vi "Least Pth Norm Complex Approximation-Compensate Channel Distortion.vi"() -> ()   [LabVIEW 2023]
doc: "Demonstrates a least pth norm complex approximation filter design. The designed filter compensates the channel distortion, both in the magnitude and phase, from some hardware devices. The goal of the compensation is to make the overall response have a flat passband magnitude response and an approximately linear phase.\n\nComplete the following steps to use this VI.\n1) Run the VI to design the bandpass finite impulse response (FIR) filter.\n2) View the graphs on the different tabs to observe the original measured channel response, designed filter magnitude, and phase response. The overall compensated channel response also is plotted.\n\n<B>Note:</B> The phase response is plotted in difference from linear phase, and the unit is in degree.\n\n3) Change the <B>Order</B>, <B>Group delay</B>, and <B>p</B>. Run the VI to redesign the filter and observe the design results."
uses:
  <vilib>/addons/Digital Filter Design/_LpNorm.llb/dfd_Lp Norm Filter Type.ctl
  <vilib>/addons/Digital Filter Design/_Objects.llb/DFD Phase Setting.ctl
  <vilib>/Utility/cursorutil.llb/Set Cursor (Icon Pict).vi
  <vilib>/addons/Digital Filter Design/Design.llb/DFD Least Pth Norm Design by IRLS.vi
  <vilib>/addons/Digital Filter Design/NI_DigFilterLicensed.lvlib
  <vilib>/Analysis/NI_AALPro.lvlib
panel:
  out "Status Str":string="Idle"
  out "Status LED":bool
  in  "?":T1(tab)
  out "Magnitude Response":cluster{dbl[], "magnitude":dbl[]}[](graph)
  out "Deviation From Linear Phase":cluster{dbl[], "magnitude":dbl[]}[](graph)
  out "Original Measured Channel Response":cluster{dbl[], dbl[]}[](graph)
  in  "p":i32=25
  in  "Order":cluster{"numerator":i32, "denominator":i32}={"numerator"=90, "denominator"=0}
  in  "Group Delay":dbl=15.0
  in  "Bandpass Specifications":T2(array[cluster])=[{"frequency point"=[{"frequency"=0.0, "magnitude"=0.0, "weight"=1.0, "phase"=0.0}]}, {"frequency point"=[{"frequency"=0.08333333333333334, "magnitude"=0.7291964977229365, "weight"=1.0, "phase"=-0.01642040201610384}, {"frequency"=0.08366700033366697, "magnitude"=0.7294776006658067, "weight"=1.0, "phase"=-0.015642400332134043}, {"frequency"=0.08400066733400066, "magnitude"=0.729821521109038, "weight"=1.0, "phase"=-0.014738419898844723}, {"frequency"=0.08433433433433435, "magnitude"=0.7302176778927697, "weight"=1.0, "phase"=-0.013743373051240626}, {"frequency"=0.08466800133466801, "magnitude"=0.7306554691620589, "weight"=1.0, "phase"=-0.01269217212432694}, {"frequency"=0.08500166833500167, "magnitude"=0.7311242586235973, "weight"=1.0, "phase"=-0.011619729453107519}, {"frequency"=0.08533533533533535, "magnitude"=0.7316133648627481, "weight"=1.0, "phase"=-0.010560957372586666}, {"frequency"=0.08566900233566904, "magnitude"=0.7321120537426865, "weight"=1.0, "phase"=-0.00955076821776979}, {"frequency"=0.0860026693360027, "magnitude"=0.7326095339186982, "weight"=1.0, "phase"=-0.00862407432366119}, {"frequency"=0.08633633633633633, "magnitude"=0.733094955508216, "weight"=1.0, "phase"=-0.007815788025265391}, {"frequency"=0.08667000333667002, "magnitude"=0.7335574119649325, "weight"=1.0, "phase"=-0.007160821643518167}, {"frequency"=0.08700367033700371, "magnitude"=0.733990132173198, "weight"=1.0, "phase"=-0.006679592999832229}, {"frequency"=0.08733733733733737, "magnitude"=0.7344025906833778, "weight"=1.0, "phase"=-0.006336255222158416}, {"frequency"=0.08767100433767103, "magnitude"=0.7348082615996662, "weight"=1.0, "phase"=-0.0060813110071700205}, {"frequency"=0.08800467133800471, "magnitude"=0.735220680155035, "weight"=1.0, "phase"=-0.005865263051539893}, {"frequency"=0.0883383383383384, "magnitude"=0.7356534427937741, "weight"=1.0, "phase"=-0.005638614051941548}, {"frequency"=0.08867200533867206, "magnitude"=0.7361202122718765, "weight"=1.0, "phase"=-0.0053518667050487245}, {"frequency"=0.08900567233900569, "magnitude"=0.7366347278394582, "weight"=1.0, "phase"=-0.004955523707534715}, {"frequency"=0.08933933933933938, "magnitude"=0.7372108205814925, "weight"=1.0, "phase"=-0.004400087756072146}, {"frequency"=0.08967300633967307, "magnitude"=0.7378624340133608, "weight"=1.0, "phase"=-0.003636061547334979}, {"frequency"=0.09000667334000673, "magnitude"=0.738603650013043, "weight"=1.0, "phase"=-0.0026139479515838726}, {"frequency"=0.09034034034034039, "magnitude"=0.7394429628053, "weight"=1.0, "phase"=-0.00130727564016353}, {"frequency"=0.09067400734067407, "magnitude"=0.7403672698363095, "weight"=1.0, "phase"=0.0002236847472032455}, {"frequency"=0.09100767434100776, "magnitude"=0.7413582649529322, "weight"=1.0, "phase"=0.0018982402282461397}, {"frequency"=0.09134134134134142, "magnitude"=0.7423974847865913, "weight"=1.0, "phase"=0.0036356978206948387}, {"frequency"=0.09167500834167505, "magnitude"=0.7434662792859068, "weight"=1.0, "phase"=0.005355364542279917}, {"frequency"=0.09200867534200874, "magnitude"=0.7445457913604945, "weight"=1.0, "phase"=0.006976547410731282}, {"frequency"=0.09234234234234243, "magnitude"=0.7456169458785842, "weight"=1.0, "phase"=0.008418553443778842}, {"frequency"=0.09267600934267609, "magnitude"=0.7466604482957828, "weight"=1.0, "phase"=0.009600689659152506}, {"frequency"=0.09300967634300975, "magnitude"=0.747656793207084, "weight"=1.0, "phase"=0.010442263074582181}, {"frequency"=0.09334334334334343, "magnitude"=0.7485862832307145, "weight"=1.0, "phase"=0.01086258136583651}, {"frequency"=0.09367701034367712, "magnitude"=0.7494340358118909, "weight"=1.0, "phase"=0.01080758126349246}, {"frequency"=0.09401067734401078, "magnitude"=0.7502033207758755, "weight"=1.0, "phase"=0.010320556929489966}, {"frequency"=0.09434434434434444, "magnitude"=0.7509016633673932, "weight"=1.0, "phase"=0.00946704597873893}, {"frequency"=0.0946780113446781, "magnitude"=0.751536690987375, "weight"=1.0, "phase"=0.008312586026149704}, {"frequency"=0.09501167834501179, "magnitude"=0.7521161195279792, "weight"=1.0, "phase"=0.006922714686632192}, {"frequency"=0.09534534534534544, "magnitude"=0.752647741160652, "weight"=1.0, "phase"=0.005362969575095633}, {"frequency"=0.0956790123456791, "magnitude"=0.7531394136376565, "weight"=1.0, "phase"=0.0036988883064501543}, {"frequency"=0.09601267934601279, "magnitude"=0.7535990511578299, "weight"=1.0, "phase"=0.0019960084956065494}, {"frequency"=0.09634634634634648, "magnitude"=0.7540346168388542, "weight"=1.0, "phase"=0.00031986775747405716}, {"frequency"=0.09668001334668014, "magnitude"=0.7544541166975602, "weight"=1.0, "phase"=-0.00126399716598935}, {"frequency"=0.0970136803470138, "magnitude"=0.7548632460642399, "weight"=1.0, "phase"=-0.0027053890336878883}, {"frequency"=0.09734734734734746, "magnitude"=0.7552593805388855, "weight"=1.0, "phase"=-0.004008541739136895}, {"frequency"=0.09768101434768114, "magnitude"=0.7556380338332156, "weight"=1.0, "phase"=-0.005189756855110916}, {"frequency"=0.0980146813480148, "magnitude"=0.7559947038644909, "weight"=1.0, "phase"=-0.006265335954384499}, {"frequency"=0.09834834834834846, "magnitude"=0.7563248750778283, "weight"=1.0, "phase"=-0.007251580609731301}, {"frequency"=0.09868201534868215, "magnitude"=0.7566240213122837, "weight"=1.0, "phase"=-0.008164792393925646}, {"frequency"=0.09901568234901584, "magnitude"=0.7568876092129782, "weight"=1.0, "phase"=-0.009021272879742526}, {"frequency"=0.0993493493493495, "magnitude"=0.7571111021899773, "weight"=1.0, "phase"=-0.009837323639955375}, {"frequency"=0.09968301634968316, "magnitude"=0.7572899649227769, "weight"=1.0, "phase"=-0.010629246247339186}, {"frequency"=0.10001668335001682, "magnitude"=0.7574196687623038, "weight"=1.0, "phase"=-0.011413341472922722}, {"frequency"=0.1003503503503505, "magnitude"=0.7574989854731671, "weight"=1.0, "phase"=-0.012198488335294577}, {"frequency"=0.10068401735068416, "magnitude"=0.7575380329833526, "weight"=1.0, "phase"=-0.012968003820737373}, {"frequency"=0.10101768435101782, "magnitude"=0.757549385635026, "weight"=1.0, "phase"=-0.013699705747336255}, {"frequency"=0.10135135135135151, "magnitude"=0.757545627611821, "weight"=1.0, "phase"=-0.014371411933176592}, {"frequency"=0.1016850183516852, "magnitude"=0.7575393458286972, "weight"=1.0, "phase"=-0.014960940196344419}, {"frequency"=0.10201868535201886, "magnitude"=0.7575431270020746, "weight"=1.0, "phase"=-0.015446108354925547}, {"frequency"=0.10235235235235252, "magnitude"=0.7575695589025218, "weight"=1.0, "phase"=-0.01580473422700579}, {"frequency"=0.10268601935268618, "magnitude"=0.7576312357911097, "weight"=1.0, "phase"=-0.01601463563067007}, {"frequency"=0.10301968635301986, "magnitude"=0.7577407680452105, "weight"=1.0, "phase"=-0.016053630384004647}, {"frequency"=0.10335335335335352, "magnitude"=0.7579107941667514, "weight"=1.0, "phase"=-0.015899538228420163}, {"frequency"=0.10368702035368718, "magnitude"=0.7581439480868885, "weight"=1.0, "phase"=-0.015540776351122831}, {"frequency"=0.10402068735402087, "magnitude"=0.7584092673045393, "weight"=1.0, "phase"=-0.015001192493993232}, {"frequency"=0.10435435435435456, "magnitude"=0.7586686932099818, "weight"=1.0, "phase"=-0.014312030150815502}, {"frequency"=0.10468802135468822, "magnitude"=0.7588840658506781, "weight"=1.0, "phase"=-0.013504532815374448}, {"frequency"=0.10502168835502187, "magnitude"=0.759017148989923, "weight"=1.0, "phase"=-0.012609943981453542}, {"frequency"=0.10535535535535553, "magnitude"=0.7590296936775417, "weight"=1.0, "phase"=-0.011659507142836922}, {"frequency"=0.10568902235568922, "magnitude"=0.7588835403489989, "weight"=1.0, "phase"=-0.010684465793309394}, {"frequency"=0.10602268935602288, "magnitude"=0.7585407591191804, "weight"=1.0, "phase"=-0.009716063426654653}, {"frequency"=0.10635635635635654, "magnitude"=0.7579638274268182, "weight"=1.0, "phase"=-0.008785543536657281}, {"frequency"=0.10669002335669023, "magnitude"=0.7571158500751093, "weight"=1.0, "phase"=-0.007924146927511755}, {"frequency"=0.10702369035702392, "magnitude"=0.7559841062871058, "weight"=1.0, "phase"=-0.007153519149495802}, {"frequency"=0.10735735735735757, "magnitude"=0.7546320301499954, "weight"=1.0, "phase"=-0.006464162750622782}, {"frequency"=0.10769102435769123, "magnitude"=0.7531378467913443, "weight"=1.0, "phase"=-0.005840273020128572}, {"frequency"=0.1080246913580249, "magnitude"=0.751578803079211, "weight"=1.0, "phase"=-0.005266045247247941}, {"frequency"=0.10835835835835858, "magnitude"=0.75003096166546, "weight"=1.0, "phase"=-0.004725674721217432}, {"frequency"=0.10869202535869224, "magnitude"=0.7485691524910209, "weight"=1.0, "phase"=-0.0042033567312727005}, {"frequency"=0.1090256923590259, "magnitude"=0.747267075522499, "weight"=1.0, "phase"=-0.003683286566649624}, {"frequency"=0.10935935935935959, "magnitude"=0.746197548757706, "weight"=1.0, "phase"=-0.003149659516583192}, {"frequency"=0.10969302635969327, "magnitude"=0.7454328970310171, "weight"=1.0, "phase"=-0.0025866708703092822}, {"frequency"=0.11002669336002693, "magnitude"=0.7450454672350842, "weight"=1.0, "phase"=-0.001978516626216953}, {"frequency"=0.1103603603603606, "magnitude"=0.7450774580732047, "weight"=1.0, "phase"=-0.0013111347269851858}, {"frequency"=0.11069402736069425, "magnitude"=0.7454750771451178, "weight"=1.0, "phase"=-0.0005759523096529051}, {"frequency"=0.11102769436102794, "magnitude"=0.7461663356684396, "weight"=1.0, "phase"=0.00023452495654474603}, {"frequency"=0.1113613613613616, "magnitude"=0.7470795280107462, "weight"=1.0, "phase"=0.0011277914023726243}, {"frequency"=0.11169502836169529, "magnitude"=0.7481427320752025, "weight"=1.0, "phase"=0.0021113413585955865}, {"frequency"=0.11202869536202895, "magnitude"=0.749283447281809, "weight"=1.0, "phase"=0.003192669155978489}, {"frequency"=0.1123623623623626, "magnitude"=0.7504283706287428, "weight"=1.0, "phase"=0.004379269125285967}, {"frequency"=0.11269602936269629, "magnitude"=0.7515033137097323, "weight"=1.0, "phase"=0.005678635597282655}, {"frequency"=0.11302969636302995, "magnitude"=0.7524332648354042, "weight"=1.0, "phase"=0.00709826290273341}, {"frequency"=0.11336336336336361, "magnitude"=0.7531426154406591, "weight"=1.0, "phase"=0.008645640535727361}, {"frequency"=0.1136970303636973, "magnitude"=0.7535820012382601, "weight"=1.0, "phase"=0.01031968524409188}, {"frequency"=0.11403069736403096, "magnitude"=0.7537834472908194, "weight"=1.0, "phase"=0.012093083021709417}, {"frequency"=0.11436436436436465, "magnitude"=0.7537950028511985, "weight"=1.0, "phase"=0.013933520165863245}, {"frequency"=0.1146980313646983, "magnitude"=0.7536650649271978, "weight"=1.0, "phase"=0.015808682973836197}, {"frequency"=0.11503169836503196, "magnitude"=0.7534421656477983, "weight"=1.0, "phase"=0.017686257742911327}, {"frequency"=0.11536536536536565, "magnitude"=0.75317482146964, "weight"=1.0, "phase"=0.019533930770371466}, {"frequency"=0.11569903236569931, "magnitude"=0.7529114448310957, "weight"=1.0, "phase"=0.021319388353499447}, {"frequency"=0.11603269936603297, "magnitude"=0.7527003182157362, "weight"=1.0, "phase"=0.023010316789578322}, {"frequency"=0.11636636636636666, "magnitude"=0.7525896302784149, "weight"=1.0, "phase"=0.024574402375890925}, {"frequency"=0.11670003336670032, "magnitude"=0.7526275620502375, "weight"=1.0, "phase"=0.025979336275783416}, {"frequency"=0.117033700367034, "magnitude"=0.7528469700766816, "weight"=1.0, "phase"=0.027199266918639387}, {"frequency"=0.11736736736736766, "magnitude"=0.7532349511268573, "weight"=1.0, "phase"=0.02822752962154551}, {"frequency"=0.11770103436770132, "magnitude"=0.7537702572793101, "weight"=1.0, "phase"=0.029061007061756072}, {"frequency"=0.11803470136803501, "magnitude"=0.7544317087878388, "weight"=1.0, "phase"=0.029696581916524467}, {"frequency"=0.11836836836836867, "magnitude"=0.7551981164450906, "weight"=1.0, "phase"=0.030131136863104535}, {"frequency"=0.11870203536870233, "magnitude"=0.7560482158426619, "weight"=1.0, "phase"=0.030361554578750116}, {"frequency"=0.11903570236903602, "magnitude"=0.7569606134289365, "weight"=1.0, "phase"=0.03038471774071483}, {"frequency"=0.11936936936936968, "magnitude"=0.75791374440808, "weight"=1.0, "phase"=0.03019750902625251}, {"frequency"=0.11970303636970336, "magnitude"=0.7588858426383042, "weight"=1.0, "phase"=0.02979681111261656}, {"frequency"=0.12003670337003702, "magnitude"=0.7598549237377591, "weight"=1.0, "phase"=0.029179516584385112}, {"frequency"=0.12037037037037068, "magnitude"=0.760799767015449, "weight"=1.0, "phase"=0.028352658384421803}, {"frequency"=0.12070403737070437, "magnitude"=0.761701802705473, "weight"=1.0, "phase"=0.027352532854794775}, {"frequency"=0.12103770437103803, "magnitude"=0.7625428113059467, "weight"=1.0, "phase"=0.02622068378784692}, {"frequency"=0.12137137137137169, "magnitude"=0.7633044390222347, "weight"=1.0, "phase"=0.02499865497592091}, {"frequency"=0.12170503837170538, "magnitude"=0.763968230946391, "weight"=1.0, "phase"=0.023727990211359407}, {"frequency"=0.12203870537203904, "magnitude"=0.7645156732675615, "weight"=1.0, "phase"=0.022450233286505084}, {"frequency"=0.12237237237237272, "magnitude"=0.7649282445346339, "weight"=1.0, "phase"=0.021206927993700386}, {"frequency"=0.12270603937270638, "magnitude"=0.7651874758978828, "weight"=1.0, "phase"=0.020039618125287983}, {"frequency"=0.12303970637304004, "magnitude"=0.7652750201436836, "weight"=1.0, "phase"=0.018989847473610544}, {"frequency"=0.12337337337337373, "magnitude"=0.7651727443448124, "weight"=1.0, "phase"=0.018099143076021118}, {"frequency"=0.12370704037370739, "magnitude"=0.7648750378917473, "weight"=1.0, "phase"=0.01739547656277618}, {"frequency"=0.12404070737404105, "magnitude"=0.7644108624232837, "weight"=1.0, "phase"=0.016868822350619705}, {"frequency"=0.12437437437437474, "magnitude"=0.7638152337984989, "weight"=1.0, "phase"=0.016502547184863436}, {"frequency"=0.1247080413747084, "magnitude"=0.7631231148491394, "weight"=1.0, "phase"=0.016280017810820002}, {"frequency"=0.12504170837504208, "magnitude"=0.7623693118813998, "weight"=1.0, "phase"=0.016184600973800922}, {"frequency"=0.12537537537537574, "magnitude"=0.7615884033021992, "weight"=1.0, "phase"=0.016199663419118826}, {"frequency"=0.1257090423757094, "magnitude"=0.7608147000421998, "weight"=1.0, "phase"=0.01630857189208479}, {"frequency"=0.12604270937604306, "magnitude"=0.7600822372374479, "weight"=1.0, "phase"=0.016494693138011662}, {"frequency"=0.12637637637637675, "magnitude"=0.7594247965425187, "weight"=1.0, "phase"=0.016741393902210966}, {"frequency"=0.12671004337671044, "magnitude"=0.7588759457608831, "weight"=1.0, "phase"=0.01703204768364519}, {"frequency"=0.1270437103770441, "magnitude"=0.7584608423530642, "weight"=1.0, "phase"=0.017354436479654956}, {"frequency"=0.12737737737737775, "magnitude"=0.7581820957925545, "weight"=1.0, "phase"=0.01770834697354684}, {"frequency"=0.1277110443777114, "magnitude"=0.758038649055317, "weight"=1.0, "phase"=0.018095590108574644}, {"frequency"=0.1280447113780451, "magnitude"=0.7580295918392452, "weight"=1.0, "phase"=0.018517976827991278}, {"frequency"=0.1283783783783788, "magnitude"=0.7581541574598288, "weight"=1.0, "phase"=0.018977318075050542}, {"frequency"=0.12871204537871245, "magnitude"=0.758411720146504, "weight"=1.0, "phase"=0.01947542479300579}, {"frequency"=0.1290457123790461, "magnitude"=0.7588017927246209, "weight"=1.0, "phase"=0.020014107925109936}, {"frequency"=0.12937937937937977, "magnitude"=0.7593240246700101, "weight"=1.0, "phase"=0.020595178414616777}, {"frequency"=0.12971304637971345, "magnitude"=0.7599782005250505, "weight"=1.0, "phase"=0.021220447204779225}, {"frequency"=0.13004671338004714, "magnitude"=0.7607642277028038, "weight"=1.0, "phase"=0.02189171669836809}, {"frequency"=0.1303803803803808, "magnitude"=0.7616762563851062, "weight"=1.0, "phase"=0.022606212271443882}, {"frequency"=0.13071404738071446, "magnitude"=0.7626928795648497, "weight"=1.0, "phase"=0.02334905001536902}, {"frequency"=0.13104771438104812, "magnitude"=0.7637899924581866, "weight"=1.0, "phase"=0.024103366347461908}, {"frequency"=0.1313813813813818, "magnitude"=0.7649432689104044, "weight"=1.0, "phase"=0.02485229768504027}, {"frequency"=0.13171504838171547, "magnitude"=0.7661281165964089, "weight"=1.0, "phase"=0.02557898044542206}, {"frequency"=0.13204871538204915, "magnitude"=0.7673196476006511, "weight"=1.0, "phase"=0.026266551045925457}, {"frequency"=0.1323823823823828, "magnitude"=0.768492664822771, "weight"=1.0, "phase"=0.026898145903868187}, {"frequency"=0.13271604938271647, "magnitude"=0.7696216647163575, "weight"=1.0, "phase"=0.027456901436568426}, {"frequency"=0.13304971638305013, "magnitude"=0.770680856886038, "weight"=1.0, "phase"=0.027925954061343905}, {"frequency"=0.13338338338338382, "magnitude"=0.7716442195449887, "weight"=1.0, "phase"=0.02828845657888923}, {"frequency"=0.1337170503837175, "magnitude"=0.7724938189234294, "weight"=1.0, "phase"=0.028534879091343557}, {"frequency"=0.13405071738405117, "magnitude"=0.7732329937236344, "weight"=1.0, "phase"=0.028674502851194772}, {"frequency"=0.13438438438438483, "magnitude"=0.773868596246044, "weight"=1.0, "phase"=0.028719590278690088}, {"frequency"=0.13471805138471848, "magnitude"=0.7744076143227507, "weight"=1.0, "phase"=0.028682403794075606}, {"frequency"=0.13505171838505217, "magnitude"=0.7748571530284708, "weight"=1.0, "phase"=0.028575205817598315}, {"frequency"=0.13538538538538586, "magnitude"=0.7752244174514789, "weight"=1.0, "phase"=0.02841025876950476}, {"frequency"=0.13571905238571952, "magnitude"=0.7755166966106241, "weight"=1.0, "phase"=0.028199825070041484}, {"frequency"=0.13605271938605318, "magnitude"=0.7757413485922225, "weight"=1.0, "phase"=0.027956167139454813}, {"frequency"=0.13638638638638684, "magnitude"=0.7759057869688721, "weight"=1.0, "phase"=0.027691547397991956}, {"frequency"=0.13672005338672052, "magnitude"=0.776017480607653, "weight"=1.0, "phase"=0.027418217720123206}, {"frequency"=0.13705372038705418, "magnitude"=0.7760884777587311, "weight"=1.0, "phase"=0.027144453398981527}, {"frequency"=0.13738738738738787, "magnitude"=0.7761422126005276, "weight"=1.0, "phase"=0.02686859494785021}, {"frequency"=0.13772105438772153, "magnitude"=0.7762038835409991, "weight"=1.0, "phase"=0.02658745687331021}, {"frequency"=0.1380547213880552, "magnitude"=0.7762987061026287, "weight"=1.0, "phase"=0.026297853681942263}, {"frequency"=0.13838838838838885, "magnitude"=0.7764519262776152, "weight"=1.0, "phase"=0.025996599880326876}, {"frequency"=0.13872205538872254, "magnitude"=0.7766888503112203, "weight"=1.0, "phase"=0.025680509975044785}, {"frequency"=0.13905572238905622, "magnitude"=0.7770348910233211, "weight"=1.0, "phase"=0.02534639847267628}, {"frequency"=0.13938938938938988, "magnitude"=0.7775156308826051, "weight"=1.0, "phase"=0.024991079879802314}, {"frequency"=0.13972305638972354, "magnitude"=0.7781569021987557, "weight"=1.0, "phase"=0.0246113687030034}, {"frequency"=0.1400567233900572, "magnitude"=0.7789848235248492, "weight"=1.0, "phase"=0.02420408589723766}, {"frequency"=0.14039039039039086, "magnitude"=0.7800061305427075, "weight"=1.0, "phase"=0.023768128762288843}, {"frequency"=0.14072405739072452, "magnitude"=0.7811795650745437, "weight"=1.0, "phase"=0.02330743640639965}, {"frequency"=0.14105772439105818, "magnitude"=0.7824563565035324, "weight"=1.0, "phase"=0.02282669841584628}, {"frequency"=0.14139139139139184, "magnitude"=0.783787198311825, "weight"=1.0, "phase"=0.02233060437690426}, {"frequency"=0.1417250583917255, "magnitude"=0.7851221459872021, "weight"=1.0, "phase"=0.02182384387584868}, {"frequency"=0.14205872539205916, "magnitude"=0.7864105772543553, "weight"=1.0, "phase"=0.021311106498955512}, {"frequency"=0.1423923923923928, "magnitude"=0.7876012167786005, "weight"=1.0, "phase"=0.020797081832500286}, {"frequency"=0.14272605939272645, "magnitude"=0.7886422275427034, "weight"=1.0, "phase"=0.020286459462758533}, {"frequency"=0.1430597263930601, "magnitude"=0.7894813707924199, "weight"=1.0, "phase"=0.019783928976005782}, {"frequency"=0.14339339339339374, "magnitude"=0.7900663336241841, "weight"=1.0, "phase"=0.019294162353024724}, {"frequency"=0.1437270603937274, "magnitude"=0.7903721297873525, "weight"=1.0, "phase"=0.01881694205332818}, {"frequency"=0.14406072739406106, "magnitude"=0.7904384644322694, "weight"=1.0, "phase"=0.018340509471393984}, {"frequency"=0.14439439439439472, "magnitude"=0.7903148153106312, "weight"=1.0, "phase"=0.01785144154599405}, {"frequency"=0.14472806139472838, "magnitude"=0.7900509258972148, "weight"=1.0, "phase"=0.017336315215900955}, {"frequency"=0.14506172839506204, "magnitude"=0.7896965978541807, "weight"=1.0, "phase"=0.016781707419886605}, {"frequency"=0.1453953953953957, "magnitude"=0.7893015459375388, "weight"=1.0, "phase"=0.01617419509672402}, {"frequency"=0.14572906239572936, "magnitude"=0.7889153156680115, "weight"=1.0, "phase"=0.01550035518518511}, {"frequency"=0.146062729396063, "magnitude"=0.7885872634877901, "weight"=1.0, "phase"=0.014746764624042452}, {"frequency"=0.14639639639639665, "magnitude"=0.7883665988554186, "weight"=1.0, "phase"=0.013900000352068176}, {"frequency"=0.1467300633967303, "magnitude"=0.7883023795503852, "weight"=1.0, "phase"=0.012946659083254985}, {"frequency"=0.14706373039706394, "magnitude"=0.7884176161425489, "weight"=1.0, "phase"=0.011878116921833382}, {"frequency"=0.1473973973973976, "magnitude"=0.7886754810078442, "weight"=1.0, "phase"=0.010696717238903197}, {"frequency"=0.14773106439773126, "magnitude"=0.7890308328248277, "weight"=1.0, "phase"=0.00940633560601567}, {"frequency"=0.14806473139806492, "magnitude"=0.789438466771787, "weight"=1.0, "phase"=0.008010847594721149}, {"frequency"=0.14839839839839858, "magnitude"=0.7898530284553761, "weight"=1.0, "phase"=0.006514128776570427}, {"frequency"=0.14873206539873224, "magnitude"=0.7902289796884825, "weight"=1.0, "phase"=0.004920054723113854}, {"frequency"=0.1490657323990659, "magnitude"=0.7905206165730275, "weight"=1.0, "phase"=0.003232501005902444}, {"frequency"=0.14939939939939956, "magnitude"=0.7906821403829216, "weight"=1.0, "phase"=0.001455343196486547}, {"frequency"=0.1497330663997332, "magnitude"=0.7906677815270303, "weight"=1.0, "phase"=-0.0004075431335828217}, {"frequency"=0.15006673340006685, "magnitude"=0.7904320804852738, "weight"=1.0, "phase"=-0.0023522401256306225}, {"frequency"=0.1504004004004005, "magnitude"=0.789952050916996, "weight"=1.0, "phase"=-0.004365865050543372}, {"frequency"=0.15073406740073414, "magnitude"=0.7892543280682364, "weight"=1.0, "phase"=-0.0064155333692217376}, {"frequency"=0.1510677344010678, "magnitude"=0.7883723804115088, "weight"=1.0, "phase"=-0.00846565416658529}, {"frequency"=0.15140140140140146, "magnitude"=0.7873396757681226, "weight"=1.0, "phase"=-0.010480636527553155}, {"frequency"=0.15173506840173512, "magnitude"=0.7861895411940636, "weight"=1.0, "phase"=-0.012424889537045125}, {"frequency"=0.15206873540206878, "magnitude"=0.7849550515057148, "weight"=1.0, "phase"=-0.014262822279980103}, {"frequency"=0.15240240240240244, "magnitude"=0.7836689463243245, "weight"=1.0, "phase"=-0.01595884384127766}, {"frequency"=0.1527360694027361, "magnitude"=0.7823635751765236, "weight"=1.0, "phase"=-0.01747736330585714}, {"frequency"=0.15306973640306976, "magnitude"=0.7810708699492893, "weight"=1.0, "phase"=-0.018782789758637897}, {"frequency"=0.1534034034034034, "magnitude"=0.7798223046093645, "weight"=1.0, "phase"=-0.01983959159961257}, {"frequency"=0.15373707040373705, "magnitude"=0.7786416306035427, "weight"=1.0, "phase"=-0.020623346504556217}, {"frequency"=0.1540707374040707, "magnitude"=0.777536480412578, "weight"=1.0, "phase"=-0.021133734673326687}, {"frequency"=0.15440440440440434, "magnitude"=0.7765123636812452, "weight"=1.0, "phase"=-0.021373594133709428}, {"frequency"=0.154738071404738, "magnitude"=0.775574775149403, "weight"=1.0, "phase"=-0.02134576291348922}, {"frequency"=0.15507173840507166, "magnitude"=0.7747292070728129, "weight"=1.0, "phase"=-0.021053079040451728}, {"frequency"=0.15540540540540532, "magnitude"=0.7739811624124456, "weight"=1.0, "phase"=-0.02049838054238151}, {"frequency"=0.15573907240573898, "magnitude"=0.7733361688179615, "weight"=1.0, "phase"=-0.019684505447064016}, {"frequency"=0.15607273940607264, "magnitude"=0.7727997934393749, "weight"=1.0, "phase"=-0.018614291782284464}, {"frequency"=0.1564064064064063, "magnitude"=0.7723776586098376, "weight"=1.0, "phase"=-0.017290577575827637}, {"frequency"=0.15674007340673995, "magnitude"=0.7720754381861281, "weight"=1.0, "phase"=-0.01571630295716475}, {"frequency"=0.1570737404070736, "magnitude"=0.7718955220278957, "weight"=1.0, "phase"=-0.013911411476722702}, {"frequency"=0.15740740740740725, "magnitude"=0.7718332930025463, "weight"=1.0, "phase"=-0.011931723652305548}, {"frequency"=0.1577410744077409, "magnitude"=0.771883344582029, "weight"=1.0, "phase"=-0.009837610392309903}, {"frequency"=0.15807474140807454, "magnitude"=0.7720403686742942, "weight"=1.0, "phase"=-0.0076894426051330456}, {"frequency"=0.1584084084084082, "magnitude"=0.7722991405081276, "weight"=1.0, "phase"=-0.0055475911991713645}, {"frequency"=0.15874207540874186, "magnitude"=0.7726545044106865, "weight"=1.0, "phase"=-0.0034724270828223602}, {"frequency"=0.15907574240907552, "magnitude"=0.773101360419999, "weight"=1.0, "phase"=-0.0015243211644822008}, {"frequency"=0.15940940940940918, "magnitude"=0.7736346516830314, "weight"=1.0, "phase"=0.0002363556474513917}, {"frequency"=0.15974307640974283, "magnitude"=0.7742493525975808, "weight"=1.0, "phase"=0.0017492324445820273}, {"frequency"=0.1600767434100765, "magnitude"=0.7749404253858766, "weight"=1.0, "phase"=0.0029541495560845288}, {"frequency"=0.16041041041041015, "magnitude"=0.7756980246918873, "weight"=1.0, "phase"=0.003822409834033591}, {"frequency"=0.16074407741074379, "magnitude"=0.7765023576223046, "weight"=1.0, "phase"=0.0043898853640069735}, {"frequency"=0.16107774441107744, "magnitude"=0.7773322689210734, "weight"=1.0, "phase"=0.004700374336808588}, {"frequency"=0.1614114114114111, "magnitude"=0.7781664297395946, "weight"=1.0, "phase"=0.004797674943243901}, {"frequency"=0.16174507841174474, "magnitude"=0.7789833289821583, "weight"=1.0, "phase"=0.004725585374116825}, {"frequency"=0.1620787454120784, "magnitude"=0.7797612764422021, "weight"=1.0, "phase"=0.004527903820232382}, {"frequency"=0.16241241241241205, "magnitude"=0.7804784179880816, "weight"=1.0, "phase"=0.004248428472394927}, {"frequency"=0.16274607941274571, "magnitude"=0.7811127630366153, "weight"=1.0, "phase"=0.003930957521409484}, {"frequency"=0.16307974641307937, "magnitude"=0.7816422245033707, "weight"=1.0, "phase"=0.0036192891580801856}, {"frequency"=0.16341341341341303, "magnitude"=0.7820447957730101, "weight"=1.0, "phase"=0.003357068641201222}, {"frequency"=0.1637470804137467, "magnitude"=0.7823151671612101, "weight"=1.0, "phase"=0.0031674603763960363}, {"frequency"=0.16408074741408035, "magnitude"=0.7824814491427057, "weight"=1.0, "phase"=0.0030327421129194843}, {"frequency"=0.16441441441441398, "magnitude"=0.7825758572218253, "weight"=1.0, "phase"=0.002930335300654674}, {"frequency"=0.16474808141474764, "magnitude"=0.782630692236983, "weight"=1.0, "phase"=0.0028376613894851577}, {"frequency"=0.1650817484150813, "magnitude"=0.7826782943728545, "weight"=1.0, "phase"=0.0027321418292947097}, {"frequency"=0.16541541541541493, "magnitude"=0.7827510238280951, "weight"=1.0, "phase"=0.0025911980699666604}, {"frequency"=0.1657490824157486, "magnitude"=0.782881268222221, "weight"=1.0, "phase"=0.002392251561384562}, {"frequency"=0.16608274941608225, "magnitude"=0.7831014768046424, "weight"=1.0, "phase"=0.0021127237534319665}, {"frequency"=0.1664164164164159, "magnitude"=0.7834442216012613, "weight"=1.0, "phase"=0.0017300360959928707}, {"frequency"=0.16675008341674957, "magnitude"=0.7839420974132115, "weight"=1.0, "phase"=0.0012217256976476687}, {"frequency"=0.16708375041708323, "magnitude"=0.7846051909938612, "weight"=1.0, "phase"=0.0005793243693956729}, {"frequency"=0.1674174174174169, "magnitude"=0.7853994173812051, "weight"=1.0, "phase"=-0.00017845628381407685}, {"frequency"=0.16775108441775055, "magnitude"=0.786285451511054, "weight"=1.0, "phase"=-0.0010297818721944907}, {"frequency"=0.16808475141808418, "magnitude"=0.7872236953163515, "weight"=1.0, "phase"=-0.001952818005959589}, {"frequency"=0.16841841841841784, "magnitude"=0.7881742040127784, "weight"=1.0, "phase"=-0.002925730295322504}, {"frequency"=0.16875208541875147, "magnitude"=0.7890966522953946, "weight"=1.0, "phase"=-0.00392668435049659}, {"frequency"=0.16908575241908513, "magnitude"=0.7899503413773119, "weight"=1.0, "phase"=-0.004933845781695201}, {"frequency"=0.1694194194194188, "magnitude"=0.7906942478624417, "weight"=1.0, "phase"=-0.005925380199132135}, {"frequency"=0.16975308641975245, "magnitude"=0.791287115327246, "weight"=1.0, "phase"=-0.0068794532130207475}, {"frequency"=0.1700867534200861, "magnitude"=0.7916877718956166, "weight"=1.0, "phase"=-0.0077743023941321265}, {"frequency"=0.17042042042041977, "magnitude"=0.791875199175099, "weight"=1.0, "phase"=-0.008596067512712136}, {"frequency"=0.17075408742075343, "magnitude"=0.7918665924579612, "weight"=1.0, "phase"=-0.009345820596954768}, {"frequency"=0.1710877544210871, "magnitude"=0.7916836670874443, "weight"=1.0, "phase"=-0.010026292763876565}, {"frequency"=0.17142142142142075, "magnitude"=0.7913483487483515, "weight"=1.0, "phase"=-0.010640215130492958}, {"frequency"=0.17175508842175438, "magnitude"=0.7908826833003659, "weight"=1.0, "phase"=-0.011190318813820044}, {"frequency"=0.17208875542208804, "magnitude"=0.7903087584550132, "weight"=1.0, "phase"=-0.011679334930873253}, {"frequency"=0.17242242242242167, "magnitude"=0.7896486376369792, "weight"=1.0, "phase"=-0.012109994598669349}, {"frequency"=0.17275608942275533, "magnitude"=0.7889243062026096, "weight"=1.0, "phase"=-0.012485028934223319}, {"frequency"=0.173089756423089, "magnitude"=0.7881576300484647, "weight"=1.0, "phase"=-0.012807169054551815}, {"frequency"=0.17342342342342265, "magnitude"=0.7873702882046637, "weight"=1.0, "phase"=-0.01307916245619778}, {"frequency"=0.1737570904237563, "magnitude"=0.7865799668699145, "weight"=1.0, "phase"=-0.013305395712733259}, {"frequency"=0.17409075742408997, "magnitude"=0.785797187968144, "weight"=1.0, "phase"=-0.013493269211688586}, {"frequency"=0.17442442442442363, "magnitude"=0.7850316370370765, "weight"=1.0, "phase"=-0.01365050706740134}, {"frequency"=0.1747580914247573, "magnitude"=0.7842929254919077, "weight"=1.0, "phase"=-0.013784833394208773}, {"frequency"=0.17509175842509092, "magnitude"=0.78359059621545, "weight"=1.0, "phase"=-0.013903972306448242}, {"frequency"=0.17542542542542458, "magnitude"=0.7829341314503409, "weight"=1.0, "phase"=-0.014015647918457108}, {"frequency"=0.17575909242575824, "magnitude"=0.7823329629570455, "weight"=1.0, "phase"=-0.014127584344572619}, {"frequency"=0.17609275942609187, "magnitude"=0.7817964844107049, "weight"=1.0, "phase"=-0.014247505699132135}, {"frequency"=0.17642642642642553, "magnitude"=0.7813340660214041, "weight"=1.0, "phase"=-0.014383136096472904}, {"frequency"=0.1767600934267592, "magnitude"=0.7809549212888665, "weight"=1.0, "phase"=-0.014542192217718353}, {"frequency"=0.17709376042709285, "magnitude"=0.7806545489148162, "weight"=1.0, "phase"=-0.014731710355687544}, {"frequency"=0.1774274274274265, "magnitude"=0.7804039618813459, "weight"=1.0, "phase"=-0.01495750933809159}, {"frequency"=0.17776109442776017, "magnitude"=0.780171729007459, "weight"=1.0, "phase"=-0.015225281606331409}, {"frequency"=0.17809476142809383, "magnitude"=0.7799265018414864, "weight"=1.0, "phase"=-0.015540719601807917}, {"frequency"=0.1784284284284275, "magnitude"=0.7796370124313223, "weight"=1.0, "phase"=-0.015909515765922144}, {"frequency"=0.17876209542876112, "magnitude"=0.7792720961989618, "weight"=1.0, "phase"=-0.01633736254007523}, {"frequency"=0.17909576242909478, "magnitude"=0.7788007397033747, "weight"=1.0, "phase"=-0.016829952365667866}, {"frequency"=0.17942942942942844, "magnitude"=0.7781921529576563, "weight"=1.0, "phase"=-0.017392977684101307}, {"frequency"=0.17976309642976207, "magnitude"=0.7774158657666472, "weight"=1.0, "phase"=-0.018032130936776358}, {"frequency"=0.18009676343009573, "magnitude"=0.7764421599476653, "weight"=1.0, "phase"=-0.018752879901885122}, {"frequency"=0.1804304304304294, "magnitude"=0.7752680846308073, "weight"=1.0, "phase"=-0.019541816438331083}, {"frequency"=0.18076409743076305, "magnitude"=0.7739364963197164, "weight"=1.0, "phase"=-0.020352659974254617}, {"frequency"=0.1810977644310967, "magnitude"=0.7724944530038845, "weight"=1.0, "phase"=-0.02113583298286492}, {"frequency"=0.18143143143143037, "magnitude"=0.7709884550783581, "weight"=1.0, "phase"=-0.02184175793737153}, {"frequency"=0.18176509843176403, "magnitude"=0.769464343942917, "weight"=1.0, "phase"=-0.022420857310983644}, {"frequency"=0.1820987654320977, "magnitude"=0.7679672565700568, "weight"=1.0, "phase"=-0.02282355357691057}, {"frequency"=0.18243243243243132, "magnitude"=0.7665416339934503, "weight"=1.0, "phase"=-0.023000269208361623}, {"frequency"=0.18276609943276498, "magnitude"=0.7652312815911121, "weight"=1.0, "phase"=-0.02290142667854622}, {"frequency"=0.18309976643309864, "magnitude"=0.7640794792196335, "weight"=1.0, "phase"=-0.022477448460673455}, {"frequency"=0.18343343343343227, "magnitude"=0.763128816455821, "weight"=1.0, "phase"=-0.021679256355123466}, {"frequency"=0.18376710043376593, "magnitude"=0.762396763376875, "weight"=1.0, "phase"=-0.02049640529040564}, {"frequency"=0.1841007674340996, "magnitude"=0.761858750809536, "weight"=1.0, "phase"=-0.018983936028781567}, {"frequency"=0.18443443443443325, "magnitude"=0.7614865763417724, "weight"=1.0, "phase"=-0.017203232636939902}, {"frequency"=0.1847681014347669, "magnitude"=0.7612523880355236, "weight"=1.0, "phase"=-0.01521567918156963}, {"frequency"=0.18510176843510057, "magnitude"=0.761128573548382, "weight"=1.0, "phase"=-0.013082659729359403}, {"frequency"=0.18543543543543423, "magnitude"=0.7610876701358569, "weight"=1.0, "phase"=-0.010865558346998205}, {"frequency"=0.18576910243576789, "magnitude"=0.7611022949262735, "weight"=1.0, "phase"=-0.008625759101174468}, {"frequency"=0.18610276943610152, "magnitude"=0.7611450951049089, "weight"=1.0, "phase"=-0.00642464605857751}, {"frequency"=0.18643643643643518, "magnitude"=0.7611887178255707, "weight"=1.0, "phase"=-0.004323603285895872}, {"frequency"=0.18677010343676884, "magnitude"=0.7612061098859204, "weight"=1.0, "phase"=-0.0023835745623049798}, {"frequency"=0.18710377043710247, "magnitude"=0.7611923755147278, "weight"=1.0, "phase"=-0.0006340398028947813}, {"frequency"=0.18743743743743613, "magnitude"=0.7611791869901544, "weight"=1.0, "phase"=0.0009474370951433331}, {"frequency"=0.1877711044377698, "magnitude"=0.7612016341731817, "weight"=1.0, "phase"=0.002388147338868829}, {"frequency"=0.18810477143810345, "magnitude"=0.7612948218792615, "weight"=1.0, "phase"=0.003715382135341061}, {"frequency"=0.1884384384384371, "magnitude"=0.7614939189492174, "weight"=1.0, "phase"=0.0049564326916193835}, {"frequency"=0.18877210543877077, "magnitude"=0.7618342398731551, "weight"=1.0, "phase"=0.00613859021476304}, {"frequency"=0.18910577243910442, "magnitude"=0.7623513593848505, "weight"=1.0, "phase"=0.007289145911831607}, {"frequency"=0.18943943943943806, "magnitude"=0.7630812608276689, "weight"=1.0, "phase"=0.008435390989884217}, {"frequency"=0.18977310643977172, "magnitude"=0.7640605196125, "weight"=1.0, "phase"=0.009604616655980336}, {"frequency"=0.19010677344010538, "magnitude"=0.7653260205824789, "weight"=1.0, "phase"=0.01082378521657823}, {"frequency"=0.19044044044043903, "magnitude"=0.7668822715457455, "weight"=1.0, "phase"=0.012098089227209119}, {"frequency"=0.19077410744077267, "magnitude"=0.7686805085527719, "weight"=1.0, "phase"=0.01339775242870167}, {"frequency"=0.19110777444110633, "magnitude"=0.7706666386269962, "weight"=1.0, "phase"=0.014689842529357566}, {"frequency"=0.19144144144143999, "magnitude"=0.7727857390054443, "weight"=1.0, "phase"=0.01594142723747838}, {"frequency"=0.19177510844177365, "magnitude"=0.7749818183568336, "weight"=1.0, "phase"=0.0171195742613659}, {"frequency"=0.1921087754421073, "magnitude"=0.7771976551248649, "weight"=1.0, "phase"=0.01819135130932159}, {"frequency"=0.19244244244244096, "magnitude"=0.7793747170298282, "weight"=1.0, "phase"=0.019123826089647245}, {"frequency"=0.19277610944277462, "magnitude"=0.7814531665522428, "weight"=1.0, "phase"=0.019884066310644544}, {"frequency"=0.19310977644310826, "magnitude"=0.7833719575077734, "weight"=1.0, "phase"=0.02043913968061506}, {"frequency"=0.19344344344344191, "magnitude"=0.7850695071072663, "weight"=1.0, "phase"=0.02075650639096871}, {"frequency"=0.19377711044377557, "magnitude"=0.7865130996553082, "weight"=1.0, "phase"=0.020827750839941817}, {"frequency"=0.19411077744410923, "magnitude"=0.7877164340277312, "weight"=1.0, "phase"=0.02068218450278858}, {"frequency"=0.19444444444444287, "magnitude"=0.7886979140195214, "weight"=1.0, "phase"=0.02035240361412316}, {"frequency"=0.19477811144477652, "magnitude"=0.7894765420990544, "weight"=1.0, "phase"=0.019871004408559934}, {"frequency"=0.19511177844511018, "magnitude"=0.790071815637584, "weight"=1.0, "phase"=0.01927058312071317}, {"frequency"=0.19544544544544384, "magnitude"=0.7905036305838448, "weight"=1.0, "phase"=0.018583735985196914}, {"frequency"=0.1957791124457775, "magnitude"=0.7907921935484516, "weight"=1.0, "phase"=0.017843059236625547}, {"frequency"=0.19611277944611116, "magnitude"=0.7909579430794995, "weight"=1.0, "phase"=0.017081149109613225}, {"frequency"=0.19644644644644482, "magnitude"=0.7910214807392825, "weight"=1.0, "phase"=0.016330601838774328}, {"frequency"=0.19678011344677845, "magnitude"=0.7910034321248022, "weight"=1.0, "phase"=0.015623727919529817}, {"frequency"=0.1971137804471121, "magnitude"=0.7909198848491026, "weight"=1.0, "phase"=0.014976488482277062}, {"frequency"=0.19744744744744577, "magnitude"=0.7907799583133622, "weight"=1.0, "phase"=0.014379949986428331}, {"frequency"=0.19778111444777943, "magnitude"=0.7905921991227813, "weight"=1.0, "phase"=0.013823088801961925}, {"frequency"=0.19811478144811306, "magnitude"=0.7903651573287301, "weight"=1.0, "phase"=0.01329488129885581}, {"frequency"=0.19844844844844672, "magnitude"=0.7901073770356786, "weight"=1.0, "phase"=0.012784303847088507}, {"frequency"=0.19878211544878038, "magnitude"=0.7898273888597787, "weight"=1.0, "phase"=0.012280332816637984}, {"frequency"=0.19911578244911404, "magnitude"=0.7895337042390476, "weight"=1.0, "phase"=0.01177194457748254}, {"frequency"=0.1994494494494477, "magnitude"=0.7892348115891015, "weight"=1.0, "phase"=0.011248115499600364}, {"frequency"=0.19978311644978136, "magnitude"=0.788939174294086, "weight"=1.0, "phase"=0.010697821952969755}, {"frequency"=0.20011678345011502, "magnitude"=0.788655244788933, "weight"=1.0, "phase"=0.010110321268279154}, {"frequency"=0.20045045045044865, "magnitude"=0.7883922131192629, "weight"=1.0, "phase"=0.009489869818689045}, {"frequency"=0.2007841174507823, "magnitude"=0.7881603753191809, "weight"=1.0, "phase"=0.00886296246810736}, {"frequency"=0.20111778445111597, "magnitude"=0.787970100399019, "weight"=1.0, "phase"=0.008257893703417785}, {"frequency"=0.20145145145144963, "magnitude"=0.7878317484848482, "weight"=1.0, "phase"=0.007702958011503891}, {"frequency"=0.20178511845178326, "magnitude"=0.7877556831411308, "weight"=1.0, "phase"=0.007226449879249475}, {"frequency"=0.20211878545211692, "magnitude"=0.7877522864234318, "weight"=1.0, "phase"=0.006856663793538442}, {"frequency"=0.20245245245245058, "magnitude"=0.7878319766862969, "weight"=1.0, "phase"=0.006621894241254145}, {"frequency"=0.20278611945278424, "magnitude"=0.7880052291896679, "weight"=1.0, "phase"=0.0065504357092806}, {"frequency"=0.2031197864531179, "magnitude"=0.7882825995686535, "weight"=1.0, "phase"=0.0066705826845014915}, {"frequency"=0.20345345345345156, "magnitude"=0.7886744834495161, "weight"=1.0, "phase"=0.007010054495130924}, {"frequency"=0.20378712045378522, "magnitude"=0.7891780764666628, "weight"=1.0, "phase"=0.007567861452006386}, {"frequency"=0.20412078745411885, "magnitude"=0.7897713733762997, "weight"=1.0, "phase"=0.008301563782258436}, {"frequency"=0.2044544544544525, "magnitude"=0.7904308015314588, "weight"=1.0, "phase"=0.009165490094484308}, {"frequency"=0.20478812145478617, "magnitude"=0.7911326715306077, "weight"=1.0, "phase"=0.010113968997281342}, {"frequency"=0.20512178845511983, "magnitude"=0.791853144261536, "weight"=1.0, "phase"=0.011101329099246882}, {"frequency"=0.20545545545545346, "magnitude"=0.7925682121202886, "weight"=1.0, "phase"=0.012081899008978159}, {"frequency"=0.20578912245578712, "magnitude"=0.7932536946422946, "weight"=1.0, "phase"=0.013010007335072737}, {"frequency"=0.20612278945612078, "magnitude"=0.7938852488130205, "weight"=1.0, "phase"=0.01383998268612785}, {"frequency"=0.20645645645645444, "magnitude"=0.7944383943186978, "weight"=1.0, "phase"=0.014526153670740838}, {"frequency"=0.2067901234567881, "magnitude"=0.794888872738692, "weight"=1.0, "phase"=0.015023255141737302}, {"frequency"=0.20712379045712176, "magnitude"=0.7952273056477532, "weight"=1.0, "phase"=0.01530501958997843}, {"frequency"=0.20745745745745542, "magnitude"=0.795465364283819, "weight"=1.0, "phase"=0.015371891060834808}, {"frequency"=0.20779112445778905, "magnitude"=0.7956164072774161, "weight"=1.0, "phase"=0.015226319012002665}, {"frequency"=0.2081247914581227, "magnitude"=0.7956938772257235, "weight"=1.0, "phase"=0.014870752901178341}, {"frequency"=0.20845845845845637, "magnitude"=0.7957112735314166, "weight"=1.0, "phase"=0.014307642186058178}, {"frequency"=0.20879212545879003, "magnitude"=0.7956821297208004, "weight"=1.0, "phase"=0.013539436324338405}, {"frequency"=0.20912579245912366, "magnitude"=0.7956199953124437, "weight"=1.0, "phase"=0.012568584773715474}, {"frequency"=0.20945945945945732, "magnitude"=0.7955384222785261, "weight"=1.0, "phase"=0.011397536991885504}, {"frequency"=0.20979312645979098, "magnitude"=0.7954509561185107, "weight"=1.0, "phase"=0.010028742436544835}, {"frequency"=0.21012679346012464, "magnitude"=0.7953710208410371, "weight"=1.0, "phase"=0.008465279155193572}, {"frequency"=0.2104604604604583, "magnitude"=0.7953071713201773, "weight"=1.0, "phase"=0.006737816887710801}, {"frequency"=0.21079412746079196, "magnitude"=0.7952613058024552, "weight"=1.0, "phase"=0.004914808304224638}, {"frequency"=0.21112779446112562, "magnitude"=0.795234843255541, "weight"=1.0, "phase"=0.00306743625693795}, {"frequency"=0.21146146146145925, "magnitude"=0.7952292049746124, "weight"=1.0, "phase"=0.00126688359805327}, {"frequency"=0.2117951284617929, "magnitude"=0.7952458153019017, "weight"=1.0, "phase"=-0.00041566682022653456}, {"frequency"=0.21212879546212657, "magnitude"=0.7952861023983617, "weight"=1.0, "phase"=-0.001909032145698708}, {"frequency"=0.21246246246246023, "magnitude"=0.7953514990681063, "weight"=1.0, "phase"=-0.0031420295261607167}, {"frequency"=0.21279612946279386, "magnitude"=0.7954434436364034, "weight"=1.0, "phase"=-0.004043476109409583}, {"frequency"=0.21312979646312752, "magnitude"=0.7955633808821183, "weight"=1.0, "phase"=-0.0045421890432427725}, {"frequency"=0.21346346346346118, "magnitude"=0.7957127638878774, "weight"=1.0, "phase"=-0.004568706918068766}, {"frequency"=0.21379713046379484, "magnitude"=0.7958930898275128, "weight"=1.0, "phase"=-0.004124619454073386}, {"frequency"=0.2141307974641285, "magnitude"=0.7961059130518888, "weight"=1.0, "phase"=-0.0033062773195537964}, {"frequency"=0.21446446446446216, "magnitude"=0.796352802194954, "weight"=1.0, "phase"=-0.002216618191444586}, {"frequency"=0.21479813146479582, "magnitude"=0.7966353381786848, "weight"=1.0, "phase"=-0.0009585797466802326}, {"frequency"=0.21513179846512945, "magnitude"=0.79695511558619, "weight"=1.0, "phase"=0.00036490033780467446}, {"frequency"=0.2154654654654631, "magnitude"=0.7973137441072607, "weight"=1.0, "phase"=0.0016508843850755461}, {"frequency"=0.21579913246579677, "magnitude"=0.7977128500588958, "weight"=1.0, "phase"=0.0027964347181977933}, {"frequency"=0.21613279946613043, "magnitude"=0.7981540779835888, "weight"=1.0, "phase"=0.003698613660236938}, {"frequency"=0.21646646646646406, "magnitude"=0.7986390923284495, "weight"=1.0, "phase"=0.00425448353425828}, {"frequency"=0.21680013346679772, "magnitude"=0.7991693623179742, "weight"=1.0, "phase"=0.004363079510092627}, {"frequency"=0.21713380046713138, "magnitude"=0.7997379357327682, "weight"=1.0, "phase"=0.004000131175572519}, {"frequency"=0.21746746746746504, "magnitude"=0.8003268476620093, "weight"=1.0, "phase"=0.0032409968801813127}, {"frequency"=0.2178011344677987, "magnitude"=0.8009172972293429, "weight"=1.0, "phase"=0.002167693331235454}, {"frequency"=0.21813480146813236, "magnitude"=0.8014903732960771, "weight"=1.0, "phase"=0.0008622372360517216}, {"frequency"=0.218468468468466, "magnitude"=0.8020270580115433, "weight"=1.0, "phase"=-0.0005933546980532167}, {"frequency"=0.21880213546879965, "magnitude"=0.8025082393775741, "weight"=1.0, "phase"=-0.0021170657637629153}, {"frequency"=0.2191358024691333, "magnitude"=0.8029147329433138, "weight"=1.0, "phase"=-0.0036268792537608174}, {"frequency"=0.21946946946946697, "magnitude"=0.803227312712601, "weight"=1.0, "phase"=-0.005040778460730255}, {"frequency"=0.21980313646980063, "magnitude"=0.8034267512935976, "weight"=1.0, "phase"=-0.006276746677354561}, {"frequency"=0.22013680347013426, "magnitude"=0.80349428797754, "weight"=1.0, "phase"=-0.007254127491303053}, {"frequency"=0.22047047047046792, "magnitude"=0.803426621219698, "weight"=1.0, "phase"=-0.007942150532348369}, {"frequency"=0.22080413747080158, "magnitude"=0.8032400036041966, "weight"=1.0, "phase"=-0.008373167629492806}, {"frequency"=0.22113780447113524, "magnitude"=0.8029520195830357, "weight"=1.0, "phase"=-0.008583584180664516}, {"frequency"=0.2214714714714689, "magnitude"=0.8025802898237334, "weight"=1.0, "phase"=-0.00860980558379143}, {"frequency"=0.22180513847180255, "magnitude"=0.8021424307605831, "weight"=1.0, "phase"=-0.00848823723680181}, {"frequency"=0.22213880547213619, "magnitude"=0.8016560218770211, "weight"=1.0, "phase"=-0.008255284537623586}, {"frequency"=0.22247247247246985, "magnitude"=0.8011385807451353, "weight"=1.0, "phase"=-0.0079473528841848}, {"frequency"=0.2228061394728035, "magnitude"=0.8006075457953579, "weight"=1.0, "phase"=-0.007600847674413491}, {"frequency"=0.22313980647313716, "magnitude"=0.8000802667507477, "weight"=1.0, "phase"=-0.007252174306237591}, {"frequency"=0.22347347347347082, "magnitude"=0.7995737037075542, "weight"=1.0, "phase"=-0.006937246314544621}, {"frequency"=0.22380714047380446, "magnitude"=0.7990943882240685, "weight"=1.0, "phase"=-0.0066749355952679945}, {"frequency"=0.22414080747413812, "magnitude"=0.7986360892668216, "weight"=1.0, "phase"=-0.006463109458333949}, {"frequency"=0.22447447447447177, "magnitude"=0.7981918236100828, "weight"=1.0, "phase"=-0.006298339884038606}, {"frequency"=0.22480814147480543, "magnitude"=0.7977546409621619, "weight"=1.0, "phase"=-0.006177198852677979}, {"frequency"=0.2251418084751391, "magnitude"=0.7973176220848711, "weight"=1.0, "phase"=-0.006096258344548078}, {"frequency"=0.22547547547547275, "magnitude"=0.796873878122211, "weight"=1.0, "phase"=-0.0060520903399451376}, {"frequency"=0.22580914247580638, "magnitude"=0.7964165511241633, "weight"=1.0, "phase"=-0.006041266819165059}, {"frequency"=0.22614280947614004, "magnitude"=0.7959388157515586, "weight"=1.0, "phase"=-0.0060603597625039085}, {"frequency"=0.2264764764764737, "magnitude"=0.7954338821472124, "weight"=1.0, "phase"=-0.006105941150257754}, {"frequency"=0.22681014347680736, "magnitude"=0.7948951221327453, "weight"=1.0, "phase"=-0.006174304429377386}, {"frequency"=0.22714381047714102, "magnitude"=0.7943199504904261, "weight"=1.0, "phase"=-0.006252612935560564}, {"frequency"=0.22747747747747465, "magnitude"=0.793710601166952, "weight"=1.0, "phase"=-0.00631706789374642}, {"frequency"=0.22781114447780831, "magnitude"=0.7930695875935979, "weight"=1.0, "phase"=-0.006343221750454375}, {"frequency"=0.22814481147814197, "magnitude"=0.7923994156952653, "weight"=1.0, "phase"=-0.006306626952203742}, {"frequency"=0.22847847847847563, "magnitude"=0.7917025820283169, "weight"=1.0, "phase"=-0.0061828359455139426}, {"frequency"=0.2288121454788093, "magnitude"=0.7909815720810333, "weight"=1.0, "phase"=-0.005947401176904288}, {"frequency"=0.22914581247914295, "magnitude"=0.7902388587359891, "weight"=1.0, "phase"=-0.005575875092894145}, {"frequency"=0.22947947947947658, "magnitude"=0.7894769008932149, "weight"=1.0, "phase"=-0.005043810140002991}, {"frequency"=0.22981314647981024, "magnitude"=0.7886981422526422, "weight"=1.0, "phase"=-0.004326758764750083}, {"frequency"=0.2301468134801439, "magnitude"=0.7879052398379439, "weight"=1.0, "phase"=-0.0034011336248392365}, {"frequency"=0.23048048048047756, "magnitude"=0.7871079464985555, "weight"=1.0, "phase"=-0.0022700598112387893}, {"frequency"=0.23081414748081122, "magnitude"=0.786324242388694, "weight"=1.0, "phase"=-0.0009679059831291803}, {"frequency"=0.23114781448114485, "magnitude"=0.7855724360400013, "weight"=1.0, "phase"=0.00046918578220989104}, {"frequency"=0.2314814814814785, "magnitude"=0.7848707010466204, "weight"=1.0, "phase"=0.00200507340749867}, {"frequency"=0.23181514848181217, "magnitude"=0.7842370953989841, "weight"=1.0, "phase"=0.00360361481545729}, {"frequency"=0.23214881548214583, "magnitude"=0.7836895890660632, "weight"=1.0, "phase"=0.005228667928806108}, {"frequency"=0.2324824824824795, "magnitude"=0.7832460997367278, "weight"=1.0, "phase"=0.006844090670265313}, {"frequency"=0.23281614948281315, "magnitude"=0.7829245366922463, "weight"=1.0, "phase"=0.008413740962555094}, {"frequency"=0.23314981648314678, "magnitude"=0.7827428528587703, "weight"=1.0, "phase"=0.009901476728395864}, {"frequency"=0.23348348348348044, "magnitude"=0.7827185585222728, "weight"=1.0, "phase"=0.011271897877984716}, {"frequency"=0.2338171504838141, "magnitude"=0.7828532281560288, "weight"=1.0, "phase"=0.012511459873088715}, {"frequency"=0.23415081748414776, "magnitude"=0.783130264000707, "weight"=1.0, "phase"=0.01363152106655996}, {"frequency"=0.23448448448448142, "magnitude"=0.7835321890880782, "weight"=1.0, "phase"=0.014644794523640148}, {"frequency"=0.23481815148481505, "magnitude"=0.7840415854238186, "weight"=1.0, "phase"=0.015563993309570978}, {"frequency"=0.2351518184851487, "magnitude"=0.7846410419487739, "weight"=1.0, "phase"=0.016401830489594038}, {"frequency"=0.23548548548548237, "magnitude"=0.7853131102628922, "weight"=1.0, "phase"=0.017171019128951137}, {"frequency"=0.23581915248581603, "magnitude"=0.7860402680401624, "weight"=1.0, "phase"=0.017884272292883807}, {"frequency"=0.2361528194861497, "magnitude"=0.7868048901387155, "weight"=1.0, "phase"=0.01855430304663397}, {"frequency"=0.23648648648648332, "magnitude"=0.7875892274718136, "weight"=1.0, "phase"=0.019193824455443043}, {"frequency"=0.23682015348681698, "magnitude"=0.7883756349515562, "weight"=1.0, "phase"=0.01981494268163303}, {"frequency"=0.23715382048715064, "magnitude"=0.7891530872814023, "weight"=1.0, "phase"=0.02041278691687981}, {"frequency"=0.2374874874874843, "magnitude"=0.7899179913898554, "weight"=1.0, "phase"=0.020963641236560415}, {"frequency"=0.23782115448781796, "magnitude"=0.7906671201573817, "weight"=1.0, "phase"=0.02144280790704617}, {"frequency"=0.23815482148815162, "magnitude"=0.7913972240904912, "weight"=1.0, "phase"=0.021825589194708506}, {"frequency"=0.23848848848848525, "magnitude"=0.7921050326857435, "weight"=1.0, "phase"=0.022087287365918862}, {"frequency"=0.2388221554888189, "magnitude"=0.792787256069966, "weight"=1.0, "phase"=0.02220320468704845}, {"frequency"=0.23915582248915257, "magnitude"=0.79344058692032, "weight"=1.0, "phase"=0.022148643424468817}, {"frequency"=0.23948948948948623, "magnitude"=0.7940617026672475, "weight"=1.0, "phase"=0.021898905844551286}, {"frequency"=0.2398231564898199, "magnitude"=0.7946472679826199, "weight"=1.0, "phase"=0.021429294213667294}, {"frequency"=0.24015682349015352, "magnitude"=0.7951941287921979, "weight"=1.0, "phase"=0.020716171356537083}, {"frequency"=0.24049049049048718, "magnitude"=0.79570421763878, "weight"=1.0, "phase"=0.019764106242861623}, {"frequency"=0.24082415749082084, "magnitude"=0.7961850020894701, "weight"=1.0, "phase"=0.01860817072136195}, {"frequency"=0.2411578244911545, "magnitude"=0.796644269275388, "weight"=1.0, "phase"=0.017284957428496672}, {"frequency"=0.24149149149148816, "magnitude"=0.7970898471171711, "weight"=1.0, "phase"=0.015831059000724845}, {"frequency"=0.2418251584918218, "magnitude"=0.7975296009128765, "weight"=1.0, "phase"=0.014283068074505245}, {"frequency"=0.24215882549215545, "magnitude"=0.7979714314617246, "weight"=1.0, "phase"=0.01267757728629676}, {"frequency"=0.2424924924924891, "magnitude"=0.798423274743098, "weight"=1.0, "phase"=0.011051179272558276}, {"frequency"=0.24282615949282277, "magnitude"=0.7988931031693413, "weight"=1.0, "phase"=0.009440466669748626}, {"frequency"=0.24315982649315643, "magnitude"=0.7993889284313372, "weight"=1.0, "phase"=0.007882032114326754}, {"frequency"=0.2434934934934901, "magnitude"=0.7999184693602905, "weight"=1.0, "phase"=0.006411799198379697}, {"frequency"=0.24382716049382372, "magnitude"=0.8004809603082511, "weight"=1.0, "phase"=0.005048755941157834}, {"frequency"=0.24416082749415738, "magnitude"=0.8010666364600212, "weight"=1.0, "phase"=0.003794047629951891}, {"frequency"=0.24449449449449104, "magnitude"=0.8016652508488061, "weight"=1.0, "phase"=0.0026479689209850665}, {"frequency"=0.2448281614948247, "magnitude"=0.8022664970065776, "weight"=1.0, "phase"=0.0016108144704806149}, {"frequency"=0.24516182849515836, "magnitude"=0.8028600068496301, "weight"=1.0, "phase"=0.0006828789346617348}, {"frequency"=0.245495495495492, "magnitude"=0.8034353512271488, "weight"=1.0, "phase"=-0.00013554303024820857}, {"frequency"=0.24582916249582565, "magnitude"=0.8039820431740577, "weight"=1.0, "phase"=-0.0008441567680262385}, {"frequency"=0.2461628294961593, "magnitude"=0.8044895439074589, "weight"=1.0, "phase"=-0.0014426676224489343}, {"frequency"=0.24649649649649297, "magnitude"=0.8049472716010082, "weight"=1.0, "phase"=-0.0019307809372931528}, {"frequency"=0.24683016349682663, "magnitude"=0.8053450452787023, "weight"=1.0, "phase"=-0.002308435341433268}, {"frequency"=0.2471638304971603, "magnitude"=0.8056831031166929, "weight"=1.0, "phase"=-0.0025811956243697587}, {"frequency"=0.24749749749749392, "magnitude"=0.8059724295337802, "weight"=1.0, "phase"=-0.002760401441128102}, {"frequency"=0.24783116449782758, "magnitude"=0.8062245500066809, "weight"=1.0, "phase"=-0.002857655479156229}, {"frequency"=0.24816483149816124, "magnitude"=0.8064510318287874, "weight"=1.0, "phase"=-0.0028845604259022384}, {"frequency"=0.2484984984984949, "magnitude"=0.8066634751072503, "weight"=1.0, "phase"=-0.002852718968814061}, {"frequency"=0.24883216549882856, "magnitude"=0.806873507072147, "weight"=1.0, "phase"=-0.0027737337953396835}, {"frequency"=0.2491658324991622, "magnitude"=0.8070927797230321, "weight"=1.0, "phase"=-0.002659207592927204}, {"frequency"=0.24949949949949585, "magnitude"=0.8073329708333372, "weight"=1.0, "phase"=-0.0025207430490244986}, {"frequency"=0.2498331664998295, "magnitude"=0.8076057883322925, "weight"=1.0, "phase"=-0.0023699428510796094}, {"frequency"=0.25016683350016317, "magnitude"=0.8079221334472395, "weight"=1.0, "phase"=-0.0022186263815095475}, {"frequency"=0.2505005005004968, "magnitude"=0.8082735093730323, "weight"=1.0, "phase"=-0.0020835970070206544}, {"frequency"=0.2508341675008305, "magnitude"=0.8086319389442, "weight"=1.0, "phase"=-0.001986642078608325}, {"frequency"=0.25116783450116414, "magnitude"=0.8089685019879004, "weight"=1.0, "phase"=-0.0019497656422370335}, {"frequency"=0.2515015015014978, "magnitude"=0.8092541845100834, "weight"=1.0, "phase"=-0.001994971743871421}, {"frequency"=0.25183516850183146, "magnitude"=0.8094599046895734, "weight"=1.0, "phase"=-0.0021442644294759616}, {"frequency"=0.25216883550216507, "magnitude"=0.8095565597855608, "weight"=1.0, "phase"=-0.002419647745015241}, {"frequency"=0.2525025025024987, "magnitude"=0.8095150939754048, "weight"=1.0, "phase"=-0.0028431257364537332}, {"frequency"=0.2528361695028324, "magnitude"=0.8093065869666897, "weight"=1.0, "phase"=-0.0034367024497561627}, {"frequency"=0.25316983650316605, "magnitude"=0.8089023629922937, "weight"=1.0, "phase"=-0.004222381930886948}, {"frequency"=0.2535035035034997, "magnitude"=0.8082758384550397, "weight"=1.0, "phase"=-0.005220500796473543}, {"frequency"=0.25383717050383336, "magnitude"=0.8074385951178474, "weight"=1.0, "phase"=-0.006414787323757054}, {"frequency"=0.254170837504167, "magnitude"=0.8064390651668445, "weight"=1.0, "phase"=-0.007753304128714222}, {"frequency"=0.2545045045045007, "magnitude"=0.8053269634350895, "weight"=1.0, "phase"=-0.00918263497383337}, {"frequency"=0.25483817150483434, "magnitude"=0.8041515934097941, "weight"=1.0, "phase"=-0.010649363621602737}, {"frequency"=0.255171838505168, "magnitude"=0.8029617417258277, "weight"=1.0, "phase"=-0.012100073834510588}, {"frequency"=0.25550550550550166, "magnitude"=0.8018056329654183, "weight"=1.0, "phase"=-0.013481349375045137}, {"frequency"=0.25583917250583527, "magnitude"=0.8007309431199011, "weight"=1.0, "phase"=-0.014739774005694706}, {"frequency"=0.2561728395061689, "magnitude"=0.7997848699969827, "weight"=1.0, "phase"=-0.015821931488947533}, {"frequency"=0.2565065065065026, "magnitude"=0.7990142590751511, "weight"=1.0, "phase"=-0.016674405587291857}, {"frequency"=0.25684017350683624, "magnitude"=0.79846355207005, "weight"=1.0, "phase"=-0.017246104648688365}, {"frequency"=0.2571738405071699, "magnitude"=0.7981304834133035, "weight"=1.0, "phase"=-0.017534697238173302}, {"frequency"=0.25750750750750356, "magnitude"=0.7979687706840544, "weight"=1.0, "phase"=-0.017584133073789948}, {"frequency"=0.2578411745078372, "magnitude"=0.797930718325627, "weight"=1.0, "phase"=-0.017440190223011076}, {"frequency"=0.2581748415081709, "magnitude"=0.7979687990609697, "weight"=1.0, "phase"=-0.0171486467533096}, {"frequency"=0.25850850850850454, "magnitude"=0.798035534851915, "weight"=1.0, "phase"=-0.016755280732158317}, {"frequency"=0.2588421755088382, "magnitude"=0.7980834345336983, "weight"=1.0, "phase"=-0.01630587022703006}, {"frequency"=0.2591758425091718, "magnitude"=0.7980649879728274, "weight"=1.0, "phase"=-0.015846193305397688}, {"frequency"=0.25950950950950546, "magnitude"=0.7979327167669699, "weight"=1.0, "phase"=-0.015422028034733998}, {"frequency"=0.2598431765098391, "magnitude"=0.7976392813934257, "weight"=1.0, "phase"=-0.015079152482511876}, {"frequency"=0.2601768435101728, "magnitude"=0.7971399063221102, "weight"=1.0, "phase"=-0.014861620979112644}, {"frequency"=0.26051051051050644, "magnitude"=0.796435605909289, "weight"=1.0, "phase"=-0.014778914362079565}, {"frequency"=0.2608441775108401, "magnitude"=0.7955694939154848, "weight"=1.0, "phase"=-0.014808543209659769}, {"frequency"=0.26117784451117376, "magnitude"=0.7945861193372915, "weight"=1.0, "phase"=-0.014926816010079225}, {"frequency"=0.2615115115115074, "magnitude"=0.793529732557056, "weight"=1.0, "phase"=-0.015110041251563955}, {"frequency"=0.2618451785118411, "magnitude"=0.7924441810832439, "weight"=1.0, "phase"=-0.01533452742234001}, {"frequency"=0.26217884551217474, "magnitude"=0.7913728546441875, "weight"=1.0, "phase"=-0.015576583010633388}, {"frequency"=0.2625125125125084, "magnitude"=0.790358678473133, "weight"=1.0, "phase"=-0.01581251650467011}, {"frequency"=0.262846179512842, "magnitude"=0.7894441534856633, "weight"=1.0, "phase"=-0.016018636392676172}, {"frequency"=0.26317984651317566, "magnitude"=0.7886714421327609, "weight"=1.0, "phase"=-0.016171251162877626}, {"frequency"=0.2635135135135093, "magnitude"=0.7880806114769983, "weight"=1.0, "phase"=-0.016248081514111917}, {"frequency"=0.263847180513843, "magnitude"=0.787675508601101, "weight"=1.0, "phase"=-0.016253954510163537}, {"frequency"=0.26418084751417664, "magnitude"=0.78742763522556, "weight"=1.0, "phase"=-0.016218116483701056}, {"frequency"=0.2645145145145103, "magnitude"=0.7873076120160948, "weight"=1.0, "phase"=-0.016170686722049882}, {"frequency"=0.26484818151484396, "magnitude"=0.787286240864081, "weight"=1.0, "phase"=-0.016141784512535423}, {"frequency"=0.2651818485151776, "magnitude"=0.7873344209074056, "weight"=1.0, "phase"=-0.016161529142483186}, {"frequency"=0.2655155155155113, "magnitude"=0.7874230863419197, "weight"=1.0, "phase"=-0.01626003989921858}, {"frequency"=0.26584918251584494, "magnitude"=0.787523165783, "weight"=1.0, "phase"=-0.016467436070067065}, {"frequency"=0.2661828495161786, "magnitude"=0.7876055630965911, "weight"=1.0, "phase"=-0.01681383694235404}, {"frequency"=0.2665165165165122, "magnitude"=0.7876411597119035, "weight"=1.0, "phase"=-0.01732936180340501}, {"frequency"=0.26685018351684586, "magnitude"=0.787601932008673, "weight"=1.0, "phase"=-0.018041901936116156}, {"frequency"=0.2671838505171795, "magnitude"=0.787479996987371, "weight"=1.0, "phase"=-0.018938392511909027}, {"frequency"=0.2675175175175132, "magnitude"=0.7872851581074207, "weight"=1.0, "phase"=-0.019969824345245704}, {"frequency"=0.26785118451784684, "magnitude"=0.7870278419489628, "weight"=1.0, "phase"=-0.02108596795364681}, {"frequency"=0.2681848515181805, "magnitude"=0.7867184813351328, "weight"=1.0, "phase"=-0.02223659385463292}, {"frequency"=0.26851851851851416, "magnitude"=0.7863675002174747, "weight"=1.0, "phase"=-0.023371472565724624}, {"frequency"=0.2688521855188478, "magnitude"=0.7859853013320492, "weight"=1.0, "phase"=-0.024440374604442566}, {"frequency"=0.2691858525191815, "magnitude"=0.785582256627723, "weight"=1.0, "phase"=-0.025393070488307287}, {"frequency"=0.26951951951951514, "magnitude"=0.7851687004559676, "weight"=1.0, "phase"=-0.026179330734839426}, {"frequency"=0.2698531865198488, "magnitude"=0.7847549255024454, "weight"=1.0, "phase"=-0.026748925861559553}, {"frequency"=0.2701868535201824, "magnitude"=0.7843504126657085, "weight"=1.0, "phase"=-0.027054044662049866}, {"frequency"=0.27052052052051606, "magnitude"=0.7839510737944899, "weight"=1.0, "phase"=-0.027089480419561357}, {"frequency"=0.2708541875208497, "magnitude"=0.7835412816584744, "weight"=1.0, "phase"=-0.026886452141173835}, {"frequency"=0.2711878545211834, "magnitude"=0.7831051032533647, "weight"=1.0, "phase"=-0.026477351838864516}, {"frequency"=0.27152152152151704, "magnitude"=0.782626680482145, "weight"=1.0, "phase"=-0.02589457152461056}, {"frequency"=0.2718551885218507, "magnitude"=0.7820902439637085, "weight"=1.0, "phase"=-0.02517050321038921}, {"frequency"=0.27218885552218436, "magnitude"=0.7814801331532968, "weight"=1.0, "phase"=-0.024337538908177615}, {"frequency"=0.272522522522518, "magnitude"=0.7807808226484416, "weight"=1.0, "phase"=-0.02342807062995301}, {"frequency"=0.2728561895228517, "magnitude"=0.7799769545154663, "weight"=1.0, "phase"=-0.022474490387692565}, {"frequency"=0.27318985652318534, "magnitude"=0.7790533764233356, "weight"=1.0, "phase"=-0.021509190193373495}, {"frequency"=0.273523523523519, "magnitude"=0.7779970900590875, "weight"=1.0, "phase"=-0.020563487654816193}, {"frequency"=0.2738571905238526, "magnitude"=0.7768274573321483, "weight"=1.0, "phase"=-0.01965054666663519}, {"frequency"=0.27419085752418626, "magnitude"=0.7755903661960779, "weight"=1.0, "phase"=-0.01876841127792587}, {"frequency"=0.2745245245245199, "magnitude"=0.774331995555423, "weight"=1.0, "phase"=-0.017914664274931817}, {"frequency"=0.2748581915248536, "magnitude"=0.7730979447359022, "weight"=1.0, "phase"=-0.01708688844389664}, {"frequency"=0.27519185852518724, "magnitude"=0.7719332374531023, "weight"=1.0, "phase"=-0.016282666571063927}, {"frequency"=0.2755255255255209, "magnitude"=0.7708823785568933, "weight"=1.0, "phase"=-0.015499581442677272}, {"frequency"=0.27585919252585456, "magnitude"=0.7699894619546176, "weight"=1.0, "phase"=-0.01473521584498027}, {"frequency"=0.2761928595261882, "magnitude"=0.7692983285242769, "weight"=1.0, "phase"=-0.013987152564216515}, {"frequency"=0.2765265265265219, "magnitude"=0.7688527734754903, "weight"=1.0, "phase"=-0.013252974386629606}, {"frequency"=0.27686019352685554, "magnitude"=0.7686939353913294, "weight"=1.0, "phase"=-0.012530084523841216}, {"frequency"=0.2771938605271892, "magnitude"=0.7688169418786767, "weight"=1.0, "phase"=-0.011812974271846882}, {"frequency"=0.2775275275275228, "magnitude"=0.7691797589825504, "weight"=1.0, "phase"=-0.011093772403774554}, {"frequency"=0.27786119452785646, "magnitude"=0.7697396076818467, "weight"=1.0, "phase"=-0.010364539504611057}, {"frequency"=0.2781948615281901, "magnitude"=0.7704538091785265, "weight"=1.0, "phase"=-0.009617336159343213}, {"frequency"=0.2785285285285238, "magnitude"=0.7712795886179741, "weight"=1.0, "phase"=-0.008844222952957847}, {"frequency"=0.27886219552885744, "magnitude"=0.7721739260287721, "weight"=1.0, "phase"=-0.008037260470441782}, {"frequency"=0.2791958625291911, "magnitude"=0.7730934545533596, "weight"=1.0, "phase"=-0.007188509296781841}, {"frequency"=0.27952952952952476, "magnitude"=0.7739944066302054, "weight"=1.0, "phase"=-0.006290030016964849}, {"frequency"=0.2798631965298584, "magnitude"=0.7748326091574061, "weight"=1.0, "phase"=-0.005333883215977535}, {"frequency"=0.2801968635301921, "magnitude"=0.7755661227482689, "weight"=1.0, "phase"=-0.004313364592320103}, {"frequency"=0.28053053053052573, "magnitude"=0.7761932161286944, "weight"=1.0, "phase"=-0.0032410030394099346}, {"frequency"=0.2808641975308594, "magnitude"=0.7767442553598047, "weight"=1.0, "phase"=-0.002144527617692852}, {"frequency"=0.28119786453119305, "magnitude"=0.7772507145543005, "weight"=1.0, "phase"=-0.0010520818664974084}, {"frequency"=0.2815315315315267, "magnitude"=0.77774425842938, "weight"=1.0, "phase"=8.190674847842472e-06}, {"frequency"=0.2818651985318604, "magnitude"=0.7782567191733372, "weight"=1.0, "phase"=0.0010081464670143349}, {"frequency"=0.28219886553219403, "magnitude"=0.7788200992037202, "weight"=1.0, "phase"=0.0019196419706735204}, {"frequency"=0.2825325325325277, "magnitude"=0.7794666001899334, "weight"=1.0, "phase"=0.0027145336464968334}, {"frequency"=0.2828661995328613, "magnitude"=0.7802286787692745, "weight"=1.0, "phase"=0.0033646779551557288}, {"frequency"=0.28319986653319495, "magnitude"=0.7811391295340694, "weight"=1.0, "phase"=0.0038419313573216374}, {"frequency"=0.2835335335335286, "magnitude"=0.782228427988426, "weight"=1.0, "phase"=0.0041201172820145016}, {"frequency"=0.2838672005338623, "magnitude"=0.7834860474028948, "weight"=1.0, "phase"=0.004202490832803829}, {"frequency"=0.28420086753419593, "magnitude"=0.7848694378107647, "weight"=1.0, "phase"=0.004114963674608792}, {"frequency"=0.2845345345345296, "magnitude"=0.7863347569040097, "weight"=1.0, "phase"=0.0038840302777852775}, {"frequency"=0.28486820153486325, "magnitude"=0.787837568471189, "weight"=1.0, "phase"=0.003536185112689161}, {"frequency"=0.2852018685351969, "magnitude"=0.7893327716898128, "weight"=1.0, "phase"=0.0030979226496763226}, {"frequency"=0.28553553553553057, "magnitude"=0.7907745809430196, "weight"=1.0, "phase"=0.0025957373591026303}, {"frequency"=0.28586920253586423, "magnitude"=0.792116558160129, "weight"=1.0, "phase"=0.002056123711323965}, {"frequency"=0.2862028695361979, "magnitude"=0.7933116996642223, "weight"=1.0, "phase"=0.0015055761766962217}, {"frequency"=0.28653653653653155, "magnitude"=0.7943125792292083, "weight"=1.0, "phase"=0.0009705892255752607}, {"frequency"=0.28687020353686515, "magnitude"=0.7950745501863961, "weight"=1.0, "phase"=0.0004769000893667802}, {"frequency"=0.2872038705371988, "magnitude"=0.7955962531429257, "weight"=1.0, "phase"=3.935233213536726e-05}, {"frequency"=0.2875375375375325, "magnitude"=0.7959092072232342, "weight"=1.0, "phase"=-0.0003353784815044447}, {"frequency"=0.28787120453786613, "magnitude"=0.7960461843532275, "weight"=1.0, "phase"=-0.0006408146830495925}, {"frequency"=0.2882048715381998, "magnitude"=0.7960402675552712, "weight"=1.0, "phase"=-0.0008704786039971241}, {"frequency"=0.28853853853853345, "magnitude"=0.7959247183651523, "weight"=1.0, "phase"=-0.0010178925758439622}, {"frequency"=0.2888722055388671, "magnitude"=0.7957328713731374, "weight"=1.0, "phase"=-0.0010765789300870993}, {"frequency"=0.28920587253920077, "magnitude"=0.7954980564385105, "weight"=1.0, "phase"=-0.0010400599982235553}, {"frequency"=0.28953953953953443, "magnitude"=0.7952535488062733, "weight"=1.0, "phase"=-0.0009018581117502811}, {"frequency"=0.2898732065398681, "magnitude"=0.7950325471304533, "weight"=1.0, "phase"=-0.0006554956021642688}, {"frequency"=0.2902068735402017, "magnitude"=0.794866733226999, "weight"=1.0, "phase"=-0.00029678114622214147}, {"frequency"=0.29054054054053535, "magnitude"=0.7947677452794643, "weight"=1.0, "phase"=0.00014683589707743805}, {"frequency"=0.290874207540869, "magnitude"=0.794732630545243, "weight"=1.0, "phase"=0.0006247999679896976}, {"frequency"=0.29120787454120267, "magnitude"=0.7947581362276677, "weight"=1.0, "phase"=0.0010860291047645187}, {"frequency"=0.29154154154153633, "magnitude"=0.7948410374601115, "weight"=1.0, "phase"=0.0014794413456518246}, {"frequency"=0.29187520854187, "magnitude"=0.794978132511882, "weight"=1.0, "phase"=0.0017539547289015384}, {"frequency"=0.29220887554220365, "magnitude"=0.7951662382791694, "weight"=1.0, "phase"=0.0018584872927635832}, {"frequency"=0.2925425425425373, "magnitude"=0.7954021860516183, "weight"=1.0, "phase"=0.0017419570754878544}, {"frequency"=0.29287620954287097, "magnitude"=0.7956828175465989, "weight"=1.0, "phase"=0.0013532821153242613}, {"frequency"=0.29320987654320463, "magnitude"=0.796004981204663, "weight"=1.0, "phase"=0.0006413804505227272}, {"frequency"=0.2935435435435383, "magnitude"=0.796365360956926, "weight"=1.0, "phase"=-0.00043958632561227895}, {"frequency"=0.29387721054387195, "magnitude"=0.796758403094847, "weight"=1.0, "phase"=-0.0018656138722938365}, {"frequency"=0.29421087754420555, "magnitude"=0.797176948030373, "weight"=1.0, "phase"=-0.0035630246919099995}, {"frequency"=0.2945445445445392, "magnitude"=0.7976137776511819, "weight"=1.0, "phase"=-0.005457079079366933}, {"frequency"=0.29487821154487287, "magnitude"=0.7980616452645849, "weight"=1.0, "phase"=-0.007473037329570831}, {"frequency"=0.29521187854520653, "magnitude"=0.7985132728862298, "weight"=1.0, "phase"=-0.009536159737427885}, {"frequency"=0.2955455455455402, "magnitude"=0.7989613498449434, "weight"=1.0, "phase"=-0.011571706597844233}, {"frequency"=0.29587921254587385, "magnitude"=0.799398532718737, "weight"=1.0, "phase"=-0.013504938205726041}, {"frequency"=0.2962128795462075, "magnitude"=0.799817446617595, "weight"=1.0, "phase"=-0.01526111485597953}, {"frequency"=0.29654654654654117, "magnitude"=0.8002106878282272, "weight"=1.0, "phase"=-0.01676549684351089}, {"frequency"=0.2968802135468748, "magnitude"=0.8005711417968938, "weight"=1.0, "phase"=-0.01794872137468076}, {"frequency"=0.2972138805472085, "magnitude"=0.8008957058383545, "weight"=1.0, "phase"=-0.01881039215904934}, {"frequency"=0.2975475475475421, "magnitude"=0.8011840699998933, "weight"=1.0, "phase"=-0.01939788025335154}, {"frequency"=0.29788121454787575, "magnitude"=0.8014359894011763, "weight"=1.0, "phase"=-0.019759513689041858}, {"frequency"=0.2982148815482094, "magnitude"=0.8016512286098065, "weight"=1.0, "phase"=-0.019943620497574782}, {"frequency"=0.29854854854854307, "magnitude"=0.8018295618400837, "weight"=1.0, "phase"=-0.01999852871040486}, {"frequency"=0.29888221554887673, "magnitude"=0.8019707731464175, "weight"=1.0, "phase"=-0.019972566358986588}, {"frequency"=0.2992158825492104, "magnitude"=0.8020746566111246, "weight"=1.0, "phase"=-0.01991406147477437}, {"frequency"=0.29954954954954405, "magnitude"=0.8021410165263513, "weight"=1.0, "phase"=-0.01987134208922281}, {"frequency"=0.2998832165498777, "magnitude"=0.8021696675698562, "weight"=1.0, "phase"=-0.019892736233786373}, {"frequency"=0.30021688355021137, "magnitude"=0.8021602962001961, "weight"=1.0, "phase"=-0.020023121208482375}, {"frequency"=0.300550550550545, "magnitude"=0.8021108849919995, "weight"=1.0, "phase"=-0.020264732571045718}, {"frequency"=0.3008842175508787, "magnitude"=0.8020182728999747, "weight"=1.0, "phase"=-0.020591045595482138}, {"frequency"=0.30121788455121234, "magnitude"=0.8018792934579897, "weight"=1.0, "phase"=-0.020974996820757152}, {"frequency"=0.30155155155154595, "magnitude"=0.8016907999884761, "weight"=1.0, "phase"=-0.02138952278583625}, {"frequency"=0.3018852185518796, "magnitude"=0.8014496693767984, "weight"=1.0, "phase"=-0.021807560029685036}, {"frequency"=0.30221888555221327, "magnitude"=0.8011528060687423, "weight"=1.0, "phase"=-0.022202045091268968}, {"frequency"=0.3025525525525469, "magnitude"=0.8007971462818304, "weight"=1.0, "phase"=-0.022545914509553622}, {"frequency"=0.3028862195528806, "magnitude"=0.8003796624198879, "weight"=1.0, "phase"=-0.022812104823504487}, {"frequency"=0.30321988655321425, "magnitude"=0.7998973676789521, "weight"=1.0, "phase"=-0.022973552572087136}, {"frequency"=0.3035535535535479, "magnitude"=0.7993484044692424, "weight"=1.0, "phase"=-0.02300593234295431}, {"frequency"=0.30388722055388157, "magnitude"=0.798743846319481, "weight"=1.0, "phase"=-0.02291753111828626}, {"frequency"=0.3042208875542152, "magnitude"=0.7981031775980644, "weight"=1.0, "phase"=-0.022738053795075652}, {"frequency"=0.30455455455454883, "magnitude"=0.7974459204798094, "weight"=1.0, "phase"=-0.02249757959296872}, {"frequency"=0.3048882215548825, "magnitude"=0.7967914739633868, "weight"=1.0, "phase"=-0.022226187731611724}, {"frequency"=0.30522188855521615, "magnitude"=0.7961591107653843, "weight"=1.0, "phase"=-0.0219539574306509}, {"frequency"=0.3055555555555498, "magnitude"=0.7955679835849636, "weight"=1.0, "phase"=-0.021710967909732592}, {"frequency"=0.30588922255588347, "magnitude"=0.7950371405861878, "weight"=1.0, "phase"=-0.021527298388503036}, {"frequency"=0.3062228895562171, "magnitude"=0.7945855499675303, "weight"=1.0, "phase"=-0.02143302808660852}, {"frequency"=0.3065565565565508, "magnitude"=0.7942321335287588, "weight"=1.0, "phase"=-0.021458236223695304}, {"frequency"=0.30689022355688444, "magnitude"=0.793994627100312, "weight"=1.0, "phase"=-0.021629642094220636}, {"frequency"=0.3072238905572181, "magnitude"=0.7938772421669302, "weight"=1.0, "phase"=-0.021935374599098834}, {"frequency"=0.30755755755755176, "magnitude"=0.7938756123024443, "weight"=1.0, "phase"=-0.022338886393190815}, {"frequency"=0.3078912245578854, "magnitude"=0.7939853337406393, "weight"=1.0, "phase"=-0.02280322866697665}, {"frequency"=0.3082248915582191, "magnitude"=0.7942020941021611, "weight"=1.0, "phase"=-0.02329145261093657}, {"frequency"=0.30855855855855274, "magnitude"=0.7945216604635416, "weight"=1.0, "phase"=-0.023766609415550588}, {"frequency"=0.30889222555888635, "magnitude"=0.7949398680471466, "weight"=1.0, "phase"=-0.024191750271298884}, {"frequency"=0.30922589255922, "magnitude"=0.795452609487442, "weight"=1.0, "phase"=-0.024529926368661525}, {"frequency"=0.30955955955955367, "magnitude"=0.7960558246343801, "weight"=1.0, "phase"=-0.02474418889811858}, {"frequency"=0.3098932265598873, "magnitude"=0.7967454908596873, "weight"=1.0, "phase"=-0.02479758905015028}, {"frequency"=0.310226893560221, "magnitude"=0.7975163883432552, "weight"=1.0, "phase"=-0.024657599601140612}, {"frequency"=0.31056056056055464, "magnitude"=0.7983496992981394, "weight"=1.0, "phase"=-0.024340684463294293}, {"frequency"=0.3108942275608883, "magnitude"=0.7992179925836054, "weight"=1.0, "phase"=-0.023893806861805256}, {"frequency"=0.31122789456122196, "magnitude"=0.800093483407075, "weight"=1.0, "phase"=-0.02336439080997743}, {"frequency"=0.3115615615615556, "magnitude"=0.800948145493649, "weight"=1.0, "phase"=-0.022799860321114696}, {"frequency"=0.3118952285618892, "magnitude"=0.8017537152463557, "weight"=1.0, "phase"=-0.02224763940852087}, {"frequency"=0.3122288955622229, "magnitude"=0.8024817157961722, "weight"=1.0, "phase"=-0.02175515208549983}, {"frequency"=0.31256256256255655, "magnitude"=0.8031035013349621, "weight"=1.0, "phase"=-0.021369822365355395}, {"frequency"=0.3128962295628902, "magnitude"=0.8035903220240056, "weight"=1.0, "phase"=-0.02113907426139161}, {"frequency"=0.31322989656322386, "magnitude"=0.8039134096083044, "weight"=1.0, "phase"=-0.021110331786912184}, {"frequency"=0.3135635635635575, "magnitude"=0.8040459817694936, "weight"=1.0, "phase"=-0.021326485543770035}, {"frequency"=0.3138972305638912, "magnitude"=0.803981761928306, "weight"=1.0, "phase"=-0.021781950002741635}, {"frequency"=0.31423089756422484, "magnitude"=0.8037270514539387, "weight"=1.0, "phase"=-0.02244176052462099}, {"frequency"=0.3145645645645585, "magnitude"=0.8032885843927187, "weight"=1.0, "phase"=-0.023270541355558505}, {"frequency"=0.31489823156489216, "magnitude"=0.8026733244879086, "weight"=1.0, "phase"=-0.024232916741704247}, {"frequency"=0.3152318985652258, "magnitude"=0.8018884346510143, "weight"=1.0, "phase"=-0.025293510929208562}, {"frequency"=0.3155655655655595, "magnitude"=0.800941247010084, "weight"=1.0, "phase"=-0.026416948164221687}, {"frequency"=0.31589923256589314, "magnitude"=0.7998392337188093, "weight"=1.0, "phase"=-0.027567852692893746}, {"frequency"=0.31623289956622674, "magnitude"=0.7985899786914168, "weight"=1.0, "phase"=-0.028710848761375085}, {"frequency"=0.3165665665665604, "magnitude"=0.797201150409008, "weight"=1.0, "phase"=-0.02981056061581594}, {"frequency"=0.31690023356689406, "magnitude"=0.7956824000505067, "weight"=1.0, "phase"=-0.03083259782644443}, {"frequency"=0.3172339005672277, "magnitude"=0.7940631636799106, "weight"=1.0, "phase"=-0.03175274207007911}, {"frequency"=0.3175675675675614, "magnitude"=0.7923841300059917, "weight"=1.0, "phase"=-0.0325527760206209}, {"frequency"=0.31790123456789504, "magnitude"=0.7906855071797899, "weight"=1.0, "phase"=-0.03321455991392408}, {"frequency"=0.3182349015682287, "magnitude"=0.7890068339785565, "weight"=1.0, "phase"=-0.03371995398584321}, {"frequency"=0.31856856856856236, "magnitude"=0.7873869834036773, "weight"=1.0, "phase"=-0.034050818472232625}, {"frequency"=0.31890223556889596, "magnitude"=0.7858642049192857, "weight"=1.0, "phase"=-0.03418901360894688}, {"frequency"=0.3192359025692296, "magnitude"=0.7844762037076847, "weight"=1.0, "phase"=-0.03411639963184032}, {"frequency"=0.3195695695695633, "magnitude"=0.78326025557872, "weight"=1.0, "phase"=-0.0338148367767675}, {"frequency"=0.31990323656989694, "magnitude"=0.7822533565729837, "weight"=1.0, "phase"=-0.033266185279582694}, {"frequency"=0.3202369035702306, "magnitude"=0.781487566801774, "weight"=1.0, "phase"=-0.03245616969868814}, {"frequency"=0.32057057057056426, "magnitude"=0.780946899213704, "weight"=1.0, "phase"=-0.03140904398644573}, {"frequency"=0.3209042375708979, "magnitude"=0.7805882087060914, "weight"=1.0, "phase"=-0.03017118634078636}, {"frequency"=0.3212379045712316, "magnitude"=0.7803684759780333, "weight"=1.0, "phase"=-0.028789238284776586}, {"frequency"=0.32157157157156524, "magnitude"=0.7802449612631662, "weight"=1.0, "phase"=-0.02730984134148312}, {"frequency"=0.3219052385718989, "magnitude"=0.7801750755315012, "weight"=1.0, "phase"=-0.025779637033972513}, {"frequency"=0.32223890557223256, "magnitude"=0.7801162986699943, "weight"=1.0, "phase"=-0.024245266885311312}, {"frequency"=0.3225725725725662, "magnitude"=0.7800261441798703, "weight"=1.0, "phase"=-0.02275337241856623}, {"frequency"=0.3229062395728999, "magnitude"=0.7798621701976673, "weight"=1.0, "phase"=-0.021350595156803875}, {"frequency"=0.32323990657323354, "magnitude"=0.7795820367027535, "weight"=1.0, "phase"=-0.020083576623090793}, {"frequency"=0.32357357357356714, "magnitude"=0.779148511002474, "weight"=1.0, "phase"=-0.018994027449671047}, {"frequency"=0.3239072405739008, "magnitude"=0.7785718336038511, "weight"=1.0, "phase"=-0.018076159552133153}, {"frequency"=0.32424090757423446, "magnitude"=0.7778886573122328, "weight"=1.0, "phase"=-0.017297639878938897}, {"frequency"=0.3245745745745681, "magnitude"=0.7771357782770665, "weight"=1.0, "phase"=-0.016625845375883408}, {"frequency"=0.3249082415749018, "magnitude"=0.7763497648055839, "weight"=1.0, "phase"=-0.016028152988761812}, {"frequency"=0.32524190857523544, "magnitude"=0.7755669096997831, "weight"=1.0, "phase"=-0.015471939663369239}, {"frequency"=0.3255755755755691, "magnitude"=0.7748232169133773, "weight"=1.0, "phase"=-0.014924582345500759}, {"frequency"=0.32590924257590276, "magnitude"=0.7741544218559434, "weight"=1.0, "phase"=-0.014353457980951556}, {"frequency"=0.32624290957623636, "magnitude"=0.7735960446872499, "weight"=1.0, "phase"=-0.013725943515516703}, {"frequency"=0.32657657657657, "magnitude"=0.7731834760895996, "weight"=1.0, "phase"=-0.013009415894991272}, {"frequency"=0.3269102435769037, "magnitude"=0.7729485347624073, "weight"=1.0, "phase"=-0.012175902446352638}, {"frequency"=0.32724391057723734, "magnitude"=0.7728900353439866, "weight"=1.0, "phase"=-0.011240724358696719}, {"frequency"=0.327577577577571, "magnitude"=0.7729890059677603, "weight"=1.0, "phase"=-0.010242748393542}, {"frequency"=0.32791124457790466, "magnitude"=0.7732264840117445, "weight"=1.0, "phase"=-0.009221076606630352}, {"frequency"=0.3282449115782383, "magnitude"=0.7735836235911808, "weight"=1.0, "phase"=-0.00821481105370353}, {"frequency"=0.328578578578572, "magnitude"=0.7740416323661691, "weight"=1.0, "phase"=-0.00726305379050346}, {"frequency"=0.32891224557890564, "magnitude"=0.774581717645417, "weight"=1.0, "phase"=-0.006404906872771954}, {"frequency"=0.3292459125792393, "magnitude"=0.7751850416287206, "weight"=1.0, "phase"=-0.005679472356250714}, {"frequency"=0.32957957957957296, "magnitude"=0.7758326857319299, "weight"=1.0, "phase"=-0.0051258522966817766}, {"frequency"=0.3299132465799066, "magnitude"=0.7765056240205382, "weight"=1.0, "phase"=-0.004783148749806843}, {"frequency"=0.3302469135802403, "magnitude"=0.7771852157689839, "weight"=1.0, "phase"=-0.004684574658285423}, {"frequency"=0.33058058058057394, "magnitude"=0.7778572884018041, "weight"=1.0, "phase"=-0.004810339319337664}, {"frequency"=0.33091424758090754, "magnitude"=0.7785100086303729, "weight"=1.0, "phase"=-0.005112602328619764}, {"frequency"=0.3312479145812412, "magnitude"=0.7791314882794296, "weight"=1.0, "phase"=-0.005543267850097067}, {"frequency"=0.33158158158157486, "magnitude"=0.7797097697583312, "weight"=1.0, "phase"=-0.006054240047734416}, {"frequency"=0.3319152485819085, "magnitude"=0.7802328373032698, "weight"=1.0, "phase"=-0.006597423085497489}, {"frequency"=0.3322489155822422, "magnitude"=0.7806886319538947, "weight"=1.0, "phase"=-0.007124721127351075}, {"frequency"=0.33258258258257584, "magnitude"=0.7810650702896508, "weight"=1.0, "phase"=-0.007588038337260294}, {"frequency"=0.3329162495829095, "magnitude"=0.7813500669293746, "weight"=1.0, "phase"=-0.00793927887919077}, {"frequency"=0.33324991658324316, "magnitude"=0.7815315607710083, "weight"=1.0, "phase"=-0.008130346917107345}, {"frequency"=0.33358358358357676, "magnitude"=0.7816000063175045, "weight"=1.0, "phase"=-0.008119137422925804}, {"frequency"=0.3339172505839104, "magnitude"=0.7815673653346963, "weight"=1.0, "phase"=-0.007915687585912212}, {"frequency"=0.3342509175842441, "magnitude"=0.7814567071430674, "weight"=1.0, "phase"=-0.007556882290225442}, {"frequency"=0.33458458458457774, "magnitude"=0.7812912233279834, "weight"=1.0, "phase"=-0.007079828301800095}, {"frequency"=0.3349182515849114, "magnitude"=0.7810940972096214, "weight"=1.0, "phase"=-0.006521632386570997}, {"frequency"=0.33525191858524506, "magnitude"=0.7808884782210688, "weight"=1.0, "phase"=-0.0059194013104728604}, {"frequency"=0.3355855855855787, "magnitude"=0.7806974700405819, "weight"=1.0, "phase"=-0.00531024183944051}, {"frequency"=0.3359192525859124, "magnitude"=0.7805441324246332, "weight"=1.0, "phase"=-0.004731260739408549}, {"frequency"=0.33625291958624604, "magnitude"=0.7804514966759302, "weight"=1.0, "phase"=-0.004219564776311913}, {"frequency"=0.3365865865865797, "magnitude"=0.7804425947020956, "weight"=1.0, "phase"=-0.003812260716085092}, {"frequency"=0.33692025358691335, "magnitude"=0.7805373641182336, "weight"=1.0, "phase"=-0.0035431081277241816}, {"frequency"=0.337253920587247, "magnitude"=0.7807294051503264, "weight"=1.0, "phase"=-0.0034176855146403895}, {"frequency"=0.3375875875875807, "magnitude"=0.7809991332973576, "weight"=1.0, "phase"=-0.0034274549834145684}, {"frequency"=0.33792125458791433, "magnitude"=0.7813268658555811, "weight"=1.0, "phase"=-0.0035637732324712568}, {"frequency"=0.33825492158824794, "magnitude"=0.7816928863890596, "weight"=1.0, "phase"=-0.003817996960235437}, {"frequency"=0.3385885885885816, "magnitude"=0.7820774203246488, "weight"=1.0, "phase"=-0.00418148286513198}, {"frequency"=0.33892225558891526, "magnitude"=0.7824606204883936, "weight"=1.0, "phase"=-0.004645587645585647}, {"frequency"=0.3392559225892489, "magnitude"=0.7828225626597378, "weight"=1.0, "phase"=-0.005201668000021309}, {"frequency"=0.3395895895895826, "magnitude"=0.783143251240194, "weight"=1.0, "phase"=-0.005841080626863948}, {"frequency"=0.33992325658991623, "magnitude"=0.7834026351319703, "weight"=1.0, "phase"=-0.006555182224538214}, {"frequency"=0.3402569235902499, "magnitude"=0.7835817043134431, "weight"=1.0, "phase"=-0.007335409923854841}, {"frequency"=0.34059059059058355, "magnitude"=0.7836701786589071, "weight"=1.0, "phase"=-0.008173856090111342}, {"frequency"=0.34092425759091716, "magnitude"=0.7836620770748305, "weight"=1.0, "phase"=-0.009062932363419818}, {"frequency"=0.3412579245912508, "magnitude"=0.7835515160485529, "weight"=1.0, "phase"=-0.009995052527485337}, {"frequency"=0.3415915915915845, "magnitude"=0.7833326960749298, "weight"=1.0, "phase"=-0.010962630366012638}, {"frequency"=0.34192525859191814, "magnitude"=0.78299991730265, "weight"=1.0, "phase"=-0.011958079662706678}, {"frequency"=0.3422589255922518, "magnitude"=0.7825475958167186, "weight"=1.0, "phase"=-0.012973814201272638}, {"frequency"=0.34259259259258545, "magnitude"=0.781970280479035, "weight"=1.0, "phase"=-0.014002247765415143}, {"frequency"=0.3429262595929191, "magnitude"=0.7812626702400012, "weight"=1.0, "phase"=-0.015035794138839376}, {"frequency"=0.3432599265932528, "magnitude"=0.7804196318252855, "weight"=1.0, "phase"=-0.01606686710525007}, {"frequency"=0.34359359359358643, "magnitude"=0.7794381568977449, "weight"=1.0, "phase"=-0.01708716727567905}, {"frequency"=0.3439272605939201, "magnitude"=0.7783306643086704, "weight"=1.0, "phase"=-0.018082772343255282}, {"frequency"=0.34426092759425375, "magnitude"=0.7771167736299263, "weight"=1.0, "phase"=-0.019037095092473977}, {"frequency"=0.3445945945945874, "magnitude"=0.7758160110732256, "weight"=1.0, "phase"=-0.01993353230565853}, {"frequency"=0.34492826159492107, "magnitude"=0.7744477187931806, "weight"=1.0, "phase"=-0.02075548076513256}, {"frequency"=0.3452619285952547, "magnitude"=0.7730310178229313, "weight"=1.0, "phase"=-0.021486337253219245}, {"frequency"=0.34559559559558833, "magnitude"=0.7715847808202824, "weight"=1.0, "phase"=-0.022109498552242313}, {"frequency"=0.345929262595922, "magnitude"=0.7701276143585247, "weight"=1.0, "phase"=-0.022608361444524938}, {"frequency"=0.34626292959625565, "magnitude"=0.7686778504517242, "weight"=1.0, "phase"=-0.02296632271239074}, {"frequency"=0.3465965965965893, "magnitude"=0.7672535469798036, "weight"=1.0, "phase"=-0.023166779138163007}, {"frequency"=0.34693026359692297, "magnitude"=0.7658708764178895, "weight"=1.0, "phase"=-0.023196276584527054}, {"frequency"=0.34726393059725663, "magnitude"=0.7645334618503643, "weight"=1.0, "phase"=-0.023065396671346328}, {"frequency"=0.3475975975975903, "magnitude"=0.7632392253057365, "weight"=1.0, "phase"=-0.022795799520230475}, {"frequency"=0.3479312645979239, "magnitude"=0.7619860972284876, "weight"=1.0, "phase"=-0.02240920440355254}, {"frequency"=0.34826493159825755, "magnitude"=0.7607720447614703, "weight"=1.0, "phase"=-0.021927330593685568}, {"frequency"=0.3485985985985912, "magnitude"=0.7595950696221663, "weight"=1.0, "phase"=-0.02137189736300249}, {"frequency"=0.3489322655989249, "magnitude"=0.7584532061104293, "weight"=1.0, "phase"=-0.020764623983876573}, {"frequency"=0.34926593259925853, "magnitude"=0.7573445192418407, "weight"=1.0, "phase"=-0.02012722972868064}, {"frequency"=0.3495995995995922, "magnitude"=0.7562671030012698, "weight"=1.0, "phase"=-0.019481433869787956}, {"frequency"=0.34993326659992585, "magnitude"=0.7552190787116486, "weight"=1.0, "phase"=-0.018848955679571344}, {"frequency"=0.3502669336002595, "magnitude"=0.7541999817706673, "weight"=1.0, "phase"=-0.018248655266936642}, {"frequency"=0.35060060060059317, "magnitude"=0.7532195906826523, "weight"=1.0, "phase"=-0.01767826173578746}, {"frequency"=0.35093426760092683, "magnitude"=0.7522921658869024, "weight"=1.0, "phase"=-0.01712603321104067}, {"frequency"=0.3512679346012605, "magnitude"=0.7514318653975536, "weight"=1.0, "phase"=-0.016580183143183547}, {"frequency"=0.35160160160159415, "magnitude"=0.7506527462481182, "weight"=1.0, "phase"=-0.01602892498270425}, {"frequency"=0.3519352686019278, "magnitude"=0.7499687928434277, "weight"=1.0, "phase"=-0.015460472180090057}, {"frequency"=0.35226893560226147, "magnitude"=0.7493939504273425, "weight"=1.0, "phase"=-0.014863038185828792}, {"frequency"=0.35260260260259507, "magnitude"=0.7489421636736201, "weight"=1.0, "phase"=-0.014224836450407952}, {"frequency"=0.35293626960292873, "magnitude"=0.7486274204640382, "weight"=1.0, "phase"=-0.013534080424315142}, {"frequency"=0.3532699366032624, "magnitude"=0.7484638009827957, "weight"=1.0, "phase"=-0.012778983558038082}, {"frequency"=0.35360360360359605, "magnitude"=0.7484613699305941, "weight"=1.0, "phase"=-0.011949959766643925}, {"frequency"=0.3539372706039297, "magnitude"=0.7486005855923463, "weight"=1.0, "phase"=-0.011053173569030794}, {"frequency"=0.35427093760426337, "magnitude"=0.748849056510132, "weight"=1.0, "phase"=-0.01010165338948743}, {"frequency"=0.35460460460459703, "magnitude"=0.7491743685834329, "weight"=1.0, "phase"=-0.0091084560524195}, {"frequency"=0.3549382716049307, "magnitude"=0.7495440580312934, "weight"=1.0, "phase"=-0.00808663838223267}, {"frequency"=0.3552719386052643, "magnitude"=0.7499255586845829, "weight"=1.0, "phase"=-0.007049257203332826}, {"frequency"=0.35560560560559795, "magnitude"=0.7502861774251359, "weight"=1.0, "phase"=-0.0060093693401255255}, {"frequency"=0.3559392726059316, "magnitude"=0.7505930980079423, "weight"=1.0, "phase"=-0.004980031617016323}, {"frequency"=0.35627293960626527, "magnitude"=0.7508134135407836, "weight"=1.0, "phase"=-0.003974300858411328}, {"frequency"=0.35660660660659893, "magnitude"=0.7509141878294303, "weight"=1.0, "phase"=-0.0030052338887159857}, {"frequency"=0.3569402736069326, "magnitude"=0.7508670925103403, "weight"=1.0, "phase"=-0.0020857722425462466}, {"frequency"=0.35727394060726625, "magnitude"=0.7506754780798954, "weight"=1.0, "phase"=-0.0012280580538748254}, {"frequency"=0.3576076076075999, "magnitude"=0.7503561963271124, "weight"=1.0, "phase"=-0.0004438947802664073}, {"frequency"=0.35794127460793357, "magnitude"=0.7499262325406921, "weight"=1.0, "phase"=0.00025491534017185735}, {"frequency"=0.35827494160826723, "magnitude"=0.7494026037860222, "weight"=1.0, "phase"=0.0008565700693331513}, {"frequency"=0.3586086086086009, "magnitude"=0.7488023129052311, "weight"=1.0, "phase"=0.0013492671691105462}, {"frequency"=0.35894227560893455, "magnitude"=0.7481423102505967, "weight"=1.0, "phase"=0.001721204401397003}, {"frequency"=0.3592759426092682, "magnitude"=0.7474394631819473, "weight"=1.0, "phase"=0.001960579528085593}, {"frequency"=0.35960960960960187, "magnitude"=0.7467105332935325, "weight"=1.0, "phase"=0.0020555903110693885}, {"frequency"=0.35994327660993547, "magnitude"=0.7459721612855907, "weight"=1.0, "phase"=0.001994434512241572}, {"frequency"=0.36027694361026913, "magnitude"=0.7452393252387072, "weight"=1.0, "phase"=0.001768322160452307}, {"frequency"=0.3606106106106028, "magnitude"=0.7445165996358999, "weight"=1.0, "phase"=0.001388700083469141}, {"frequency"=0.36094427761093645, "magnitude"=0.7438042957737243, "weight"=1.0, "phase"=0.0008753491370255828}, {"frequency"=0.3612779446112701, "magnitude"=0.7431027099921951, "weight"=1.0, "phase"=0.0002480760593387421}, {"frequency"=0.36161161161160377, "magnitude"=0.7424121369773851, "weight"=1.0, "phase"=-0.0004733124113742715}, {"frequency"=0.3619452786119374, "magnitude"=0.7417328698583311, "weight"=1.0, "phase"=-0.0012690095368963483}, {"frequency"=0.3622789456122711, "magnitude"=0.7410652003058701, "weight"=1.0, "phase"=-0.0021192085790103787}, {"frequency"=0.3626126126126047, "magnitude"=0.7404094186333958, "weight"=1.0, "phase"=-0.003004102799499253}, {"frequency"=0.36294627961293835, "magnitude"=0.7397658138995313, "weight"=1.0, "phase"=-0.0039038854601459727}, {"frequency"=0.363279946613272, "magnitude"=0.7391346740127098, "weight"=1.0, "phase"=-0.004798749822733539}, {"frequency"=0.36361361361360567, "magnitude"=0.7385180368868393, "weight"=1.0, "phase"=-0.005669456569468712}, {"frequency"=0.36394728061393933, "magnitude"=0.7379293096323107, "weight"=1.0, "phase"=-0.006500460466590474}, {"frequency"=0.364280947614273, "magnitude"=0.7373863672762622, "weight"=1.0, "phase"=-0.007277694906522192}, {"frequency"=0.36461461461460665, "magnitude"=0.7369070044849183, "weight"=1.0, "phase"=-0.007987097202960203}, {"frequency"=0.3649482816149403, "magnitude"=0.7365089500987959, "weight"=1.0, "phase"=-0.008614604669600845}, {"frequency"=0.36528194861527397, "magnitude"=0.7362099022661588, "weight"=1.0, "phase"=-0.009146154620140345}, {"frequency"=0.3656156156156076, "magnitude"=0.7360275720484486, "weight"=1.0, "phase"=-0.009567684368275153}, {"frequency"=0.3659492826159413, "magnitude"=0.7359797355724128, "weight"=1.0, "phase"=-0.009865131227701607}, {"frequency"=0.36628294961627494, "magnitude"=0.7360842949008399, "weight"=1.0, "phase"=-0.010024432512115933}, {"frequency"=0.3666166166166086, "magnitude"=0.7363593479093301, "weight"=1.0, "phase"=-0.01003152553521447}, {"frequency"=0.36695028361694226, "magnitude"=0.7368165258635907, "weight"=1.0, "phase"=-0.009878303786250764}, {"frequency"=0.36728395061727587, "magnitude"=0.7374251633828892, "weight"=1.0, "phase"=-0.009594244185876954}, {"frequency"=0.3676176176176095, "magnitude"=0.7381379970591287, "weight"=1.0, "phase"=-0.009223443137964527}, {"frequency"=0.3679512846179432, "magnitude"=0.7389074780888205, "weight"=1.0, "phase"=-0.008810029779285022}, {"frequency"=0.36828495161827685, "magnitude"=0.7396857045835238, "weight"=1.0, "phase"=-0.008398133246610096}, {"frequency"=0.3686186186186105, "magnitude"=0.7404243782253678, "weight"=1.0, "phase"=-0.0080318826767114}, {"frequency"=0.36895228561894416, "magnitude"=0.7410748234828561, "weight"=1.0, "phase"=-0.007755407206360809}, {"frequency"=0.3692859526192778, "magnitude"=0.7415880706681899, "weight"=1.0, "phase"=-0.007612835972329979}, {"frequency"=0.3696196196196115, "magnitude"=0.7419150038392045, "weight"=1.0, "phase"=-0.007648298111390561}, {"frequency"=0.3699532866199451, "magnitude"=0.7420065739120744, "weight"=1.0, "phase"=-0.007905922760314099}, {"frequency"=0.37028695362027875, "magnitude"=0.7418230039512521, "weight"=1.0, "phase"=-0.008417671105371949}, {"frequency"=0.3706206206206124, "magnitude"=0.7413796924509594, "weight"=1.0, "phase"=-0.009141075324075598}, {"frequency"=0.37095428762094607, "magnitude"=0.7407131113617984, "weight"=1.0, "phase"=-0.01000553516749203}, {"frequency"=0.3712879546212797, "magnitude"=0.7398599632018287, "weight"=1.0, "phase"=-0.010940397893109188}, {"frequency"=0.3716216216216134, "magnitude"=0.7388569417298856, "weight"=1.0, "phase"=-0.011875010758414795}, {"frequency"=0.37195528862194704, "magnitude"=0.7377405674560833, "weight"=1.0, "phase"=-0.012738721020896682}, {"frequency"=0.3722889556222807, "magnitude"=0.7365470598262861, "weight"=1.0, "phase"=-0.013460875938042571}, {"frequency"=0.37262262262261436, "magnitude"=0.7353122458476886, "weight"=1.0, "phase"=-0.013970822767340185}, {"frequency"=0.372956289622948, "magnitude"=0.7340715044731987, "weight"=1.0, "phase"=-0.014197908766277467}, {"frequency"=0.3732899566232817, "magnitude"=0.7328597457656698, "weight"=1.0, "phase"=-0.014071481192341917}, {"frequency"=0.37362362362361534, "magnitude"=0.7317077196809088, "weight"=1.0, "phase"=-0.013537085207094512}, {"frequency"=0.373957290623949, "magnitude"=0.730623906236164, "weight"=1.0, "phase"=-0.012636326140704535}, {"frequency"=0.3742909576242826, "magnitude"=0.7296086943752991, "weight"=1.0, "phase"=-0.01144608563949423}, {"frequency"=0.37462462462461626, "magnitude"=0.7286624897836687, "weight"=1.0, "phase"=-0.010043299391749638}, {"frequency"=0.3749582916249499, "magnitude"=0.7277857283577627, "weight"=1.0, "phase"=-0.008504903085757132}, {"frequency"=0.3752919586252836, "magnitude"=0.7269788773215684, "weight"=1.0, "phase"=-0.006907832409802417}, {"frequency"=0.37562562562561724, "magnitude"=0.7262424363896712, "weight"=1.0, "phase"=-0.005329023052171644}, {"frequency"=0.3759592926259509, "magnitude"=0.7255769389804267, "weight"=1.0, "phase"=-0.003845410701150964}, {"frequency"=0.37629295962628456, "magnitude"=0.724982953482734, "weight"=1.0, "phase"=-0.0025339310450263053}, {"frequency"=0.37662662662661817, "magnitude"=0.7244610845801335, "weight"=1.0, "phase"=-0.001471519772083707}, {"frequency"=0.3769602936269518, "magnitude"=0.7240106706222252, "weight"=1.0, "phase"=-0.000720154342202739}, {"frequency"=0.3772939606272855, "magnitude"=0.7236236037881801, "weight"=1.0, "phase"=-0.00025579537795616947}, {"frequency"=0.37762762762761914, "magnitude"=0.7232891764661945, "weight"=1.0, "phase"=-2.371721891925027e-05}, {"frequency"=0.3779612946279528, "magnitude"=0.7229967431377646, "weight"=1.0, "phase"=3.0843724725615473e-05}, {"frequency"=0.37829496162828646, "magnitude"=0.7227357097546858, "weight"=1.0, "phase"=-3.7348957204641486e-05}, {"frequency"=0.3786286286286201, "magnitude"=0.7224955229701152, "weight"=1.0, "phase"=-0.00017353167489275734}, {"frequency"=0.3789622956289538, "magnitude"=0.7222656624900043, "weight"=1.0, "phase"=-0.00032294083852135724}, {"frequency"=0.37929596262928744, "magnitude"=0.7220356365119134, "weight"=1.0, "phase"=-0.00043081285827339943}, {"frequency"=0.3796296296296211, "magnitude"=0.7217949802257475, "weight"=1.0, "phase"=-0.0004423841443315091}, {"frequency"=0.37996329662995476, "magnitude"=0.7215332573546965, "weight"=1.0, "phase"=-0.0003028911068786444}, {"frequency"=0.3802969636302884, "magnitude"=0.7212421692831072, "weight"=1.0, "phase"=3.057043469989473e-05}, {"frequency"=0.3806306306306221, "magnitude"=0.7209251763483925, "weight"=1.0, "phase"=0.0005347684219406679}, {"frequency"=0.38096429763095574, "magnitude"=0.7205897925865037, "weight"=1.0, "phase"=0.001163553255076888}, {"frequency"=0.3812979646312894, "magnitude"=0.7202435119469616, "weight"=1.0, "phase"=0.0018707529434658365}, {"frequency"=0.38163163163162306, "magnitude"=0.7198938013057586, "weight"=1.0, "phase"=0.0026101954964644625}, {"frequency"=0.3819652986319567, "magnitude"=0.7195480990139766, "weight"=1.0, "phase"=0.0033357089234297144}, {"frequency"=0.3822989656322903, "magnitude"=0.7192138149906843, "weight"=1.0, "phase"=0.004001121233718874}, {"frequency"=0.382632632632624, "magnitude"=0.7188983323448142, "weight"=1.0, "phase"=0.004560260436688668}, {"frequency"=0.38296629963295764, "magnitude"=0.7186090105114931, "weight"=1.0, "phase"=0.004966954541696378}, {"frequency"=0.3832999666332913, "magnitude"=0.7183531898903686, "weight"=1.0, "phase"=0.005175031558099064}, {"frequency"=0.38363363363362496, "magnitude"=0.7181370874309309, "weight"=1.0, "phase"=0.005147963887524476}, {"frequency"=0.38396730063395856, "magnitude"=0.7179609130907881, "weight"=1.0, "phase"=0.004901388319428879}, {"frequency"=0.3843009676342922, "magnitude"=0.7178228698063137, "weight"=1.0, "phase"=0.004468497347720479}, {"frequency"=0.3846346346346259, "magnitude"=0.7177211742196434, "weight"=1.0, "phase"=0.0038824966959258855}, {"frequency"=0.38496830163495954, "magnitude"=0.7176540563623296, "weight"=1.0, "phase"=0.003176592087572372}, {"frequency"=0.3853019686352932, "magnitude"=0.7176197579128354, "weight"=1.0, "phase"=0.0023839892461869905}, {"frequency"=0.38563563563562686, "magnitude"=0.7176165305491987, "weight"=1.0, "phase"=0.0015378938952970156}, {"frequency"=0.3859693026359605, "magnitude"=0.7176426343942607, "weight"=1.0, "phase"=0.0006715117584290553}, {"frequency"=0.3863029696362942, "magnitude"=0.7176963365511857, "weight"=1.0, "phase"=-0.00018195144088939408}, {"frequency"=0.38663663663662784, "magnitude"=0.7177759097273217, "weight"=1.0, "phase"=-0.0009892899791317245}, {"frequency"=0.3869703036369615, "magnitude"=0.7178774949134461, "weight"=1.0, "phase"=-0.0017226853149978627}, {"frequency"=0.38730397063729516, "magnitude"=0.7179860231314897, "weight"=1.0, "phase"=-0.0023825825925238853}, {"frequency"=0.3876376376376288, "magnitude"=0.7180827441273713, "weight"=1.0, "phase"=-0.0029786641055171703}, {"frequency"=0.3879713046379625, "magnitude"=0.7181488862809862, "weight"=1.0, "phase"=-0.0035206173593120837}, {"frequency"=0.38830497163829614, "magnitude"=0.7181656697458484, "weight"=1.0, "phase"=-0.00401812985924388}, {"frequency"=0.3886386386386298, "magnitude"=0.7181143273432317, "weight"=1.0, "phase"=-0.00448088911064648}, {"frequency"=0.38897230563896346, "magnitude"=0.7179761352528888, "weight"=1.0, "phase"=-0.0049185826188551385}, {"frequency"=0.38930597263929706, "magnitude"=0.7177324534200802, "weight"=1.0, "phase"=-0.005340897889203777}, {"frequency"=0.3896396396396307, "magnitude"=0.7173647755209652, "weight"=1.0, "phase"=-0.005757522427027872}, {"frequency"=0.3899733066399644, "magnitude"=0.7168547882303534, "weight"=1.0, "phase"=-0.006178143737661346}, {"frequency"=0.39030697364029804, "magnitude"=0.7161887581494313, "weight"=1.0, "phase"=-0.006606968320002071}, {"frequency"=0.3906406406406317, "magnitude"=0.7153751788489952, "weight"=1.0, "phase"=-0.00702030706658241}, {"frequency"=0.39097430764096536, "magnitude"=0.714429602379506, "weight"=1.0, "phase"=-0.007385618461164478}, {"frequency"=0.39130797464129896, "magnitude"=0.7133675845643632, "weight"=1.0, "phase"=-0.00767035738365851}, {"frequency"=0.3916416416416326, "magnitude"=0.7122046294681444, "weight"=1.0, "phase"=-0.007841978713976294}, {"frequency"=0.3919753086419663, "magnitude"=0.7109561435655116, "weight"=1.0, "phase"=-0.007867937332028951}, {"frequency"=0.39230897564229994, "magnitude"=0.7096373967938325, "weight"=1.0, "phase"=-0.007715688117726938}, {"frequency"=0.3926426426426336, "magnitude"=0.7082634904412454, "weight"=1.0, "phase"=-0.007352685950981819}, {"frequency"=0.39297630964296726, "magnitude"=0.706849331758541, "weight"=1.0, "phase"=-0.0067463857117042725}, {"frequency"=0.3933099766433009, "magnitude"=0.705409615132744, "weight"=1.0, "phase"=-0.005864242279805643}, {"frequency"=0.3936436436436346, "magnitude"=0.7039598344891148, "weight"=1.0, "phase"=-0.004684871014712488}, {"frequency"=0.39397731064396824, "magnitude"=0.7025202749933471, "weight"=1.0, "phase"=-0.0032419937573047175}, {"frequency"=0.3943109776443019, "magnitude"=0.701112438831943, "weight"=1.0, "phase"=-0.00158631082335714}, {"frequency"=0.39464464464463556, "magnitude"=0.6997574883004565, "weight"=1.0, "phase"=0.0002314727122183502}, {"frequency"=0.3949783116449692, "magnitude"=0.6984762727083826, "weight"=1.0, "phase"=0.0021606517745105247}, {"frequency"=0.3953119786453029, "magnitude"=0.6972893679598952, "weight"=1.0, "phase"=0.004150521288607489}, {"frequency"=0.39564564564563653, "magnitude"=0.6962171279668627, "weight"=1.0, "phase"=0.00615037617959846}, {"frequency"=0.3959793126459702, "magnitude"=0.6952797476053894, "weight"=1.0, "phase"=0.008109511372571543}, {"frequency"=0.39631297964630385, "magnitude"=0.694497337070075, "weight"=1.0, "phase"=0.009977221792615065}, {"frequency"=0.39664664664663746, "magnitude"=0.6938900076497287, "weight"=1.0, "phase"=0.011702802364818243}, {"frequency"=0.3969803136469711, "magnitude"=0.6934725230082226, "weight"=1.0, "phase"=0.013247631585686426}, {"frequency"=0.3973139806473048, "magnitude"=0.693233794251522, "weight"=1.0, "phase"=0.014630976269690121}, {"frequency"=0.39764764764763844, "magnitude"=0.6931552526044272, "weight"=1.0, "phase"=0.015889417899883185}, {"frequency"=0.3979813146479721, "magnitude"=0.6932185844636953, "weight"=1.0, "phase"=0.017059541101750675}, {"frequency"=0.39831498164830575, "magnitude"=0.6934056530661303, "weight"=1.0, "phase"=0.018177930500775652}, {"frequency"=0.39864864864863936, "magnitude"=0.6936984288826531, "weight"=1.0, "phase"=0.019281170722443175}, {"frequency"=0.398982315648973, "magnitude"=0.6940789297480731, "weight"=1.0, "phase"=0.020405846392236526}, {"frequency"=0.3993159826493067, "magnitude"=0.6945291704620156, "weight"=1.0, "phase"=0.021588542135640543}, {"frequency"=0.39964964964964034, "magnitude"=0.69503112171761, "weight"=1.0, "phase"=0.02286584257813895}, {"frequency"=0.399983316649974, "magnitude"=0.6955666783145382, "weight"=1.0, "phase"=0.02427433234521592}, {"frequency"=0.40031698365030766, "magnitude"=0.696118984510251, "weight"=1.0, "phase"=0.02583926184282559}, {"frequency"=0.4006506506506413, "magnitude"=0.6966773568079374, "weight"=1.0, "phase"=0.027533196111521274}, {"frequency"=0.400984317650975, "magnitude"=0.6972328686849601, "weight"=1.0, "phase"=0.029313403374505498}, {"frequency"=0.40131798465130863, "magnitude"=0.6977765369184067, "weight"=1.0, "phase"=0.031137150202520836}, {"frequency"=0.4016516516516423, "magnitude"=0.6982993231733432, "weight"=1.0, "phase"=0.03296170316631142}, {"frequency"=0.40198531865197595, "magnitude"=0.6987921381299987, "weight"=1.0, "phase"=0.03474432883662004}, {"frequency"=0.4023189856523096, "magnitude"=0.6992458479878472, "weight"=1.0, "phase"=0.03644229378419017}, {"frequency"=0.4026526526526433, "magnitude"=0.6996512833750368, "weight"=1.0, "phase"=0.03801286457976483}, {"frequency"=0.40298631965297693, "magnitude"=0.699999250683243, "weight"=1.0, "phase"=0.03941330779408769}, {"frequency"=0.4033199866533106, "magnitude"=0.7002805458369418, "weight"=1.0, "phase"=0.040600889997901346}, {"frequency"=0.40365365365364425, "magnitude"=0.7004883053599285, "weight"=1.0, "phase"=0.04154652278519455}, {"frequency"=0.40398732065397785, "magnitude"=0.7006262288376911, "weight"=1.0, "phase"=0.0422826634772735}, {"frequency"=0.4043209876543115, "magnitude"=0.7007010348728987, "weight"=1.0, "phase"=0.042859113894034406}, {"frequency"=0.4046546546546452, "magnitude"=0.7007194847182106, "weight"=1.0, "phase"=0.043325676842426386}, {"frequency"=0.40498832165497883, "magnitude"=0.7006883705671044, "weight"=1.0, "phase"=0.043732155129398764}, {"frequency"=0.4053219886553125, "magnitude"=0.7006145052860849, "weight"=1.0, "phase"=0.04412835156190065}, {"frequency"=0.4056556556556461, "magnitude"=0.700504713444939, "weight"=1.0, "phase"=0.04456406894688092}, {"frequency"=0.40598932265597976, "magnitude"=0.7003658236627133, "weight"=1.0, "phase"=0.04508911009128935}, {"frequency"=0.4063229896563134, "magnitude"=0.7002046622803146, "weight"=1.0, "phase"=0.04575327780207461}, {"frequency"=0.4066566566566471, "magnitude"=0.7000280483649342, "weight"=1.0, "phase"=0.04660637488618624}, {"frequency"=0.40699032365698073, "magnitude"=0.699840795979014, "weight"=1.0, "phase"=0.04768440192669532}, {"frequency"=0.4073239906573144, "magnitude"=0.6996389873547426, "weight"=1.0, "phase"=0.04896294851447203}, {"frequency"=0.40765765765764805, "magnitude"=0.6994163309936104, "weight"=1.0, "phase"=0.05040108071875915}, {"frequency"=0.4079913246579817, "magnitude"=0.699166554493041, "weight"=1.0, "phase"=0.05195786420048254}, {"frequency"=0.4083249916583154, "magnitude"=0.6988834089001588, "weight"=1.0, "phase"=0.05359236462056782}, {"frequency"=0.40865865865864903, "magnitude"=0.6985606741133112, "weight"=1.0, "phase"=0.055263647639941516}, {"frequency"=0.4089923256589827, "magnitude"=0.698192165374283, "weight"=1.0, "phase"=0.05693077891952858}, {"frequency"=0.40932599265931635, "magnitude"=0.6977717408307085, "weight"=1.0, "phase"=0.05855282412025575}, {"frequency"=0.40965965965965, "magnitude"=0.6972933101430164, "weight"=1.0, "phase"=0.06008884890304844}, {"frequency"=0.40999332665998367, "magnitude"=0.6967508441043414, "weight"=1.0, "phase"=0.06149791892883272}, {"frequency"=0.41032699366031733, "magnitude"=0.696143999621372, "weight"=1.0, "phase"=0.06274992345379782}, {"frequency"=0.410660660660651, "magnitude"=0.6954962746010847, "weight"=1.0, "phase"=0.06386072393130027}, {"frequency"=0.41099432766098465, "magnitude"=0.6948373216394257, "weight"=1.0, "phase"=0.06485838521159093}, {"frequency"=0.41132799466131825, "magnitude"=0.6941965753182656, "weight"=1.0, "phase"=0.06577097223691886}, {"frequency"=0.4116616616616519, "magnitude"=0.6936032555815471, "weight"=1.0, "phase"=0.06662654994953399}, {"frequency"=0.41199532866198557, "magnitude"=0.6930863958373339, "weight"=1.0, "phase"=0.06745318329168559}, {"frequency"=0.41232899566231923, "magnitude"=0.6926748953240792, "weight"=1.0, "phase"=0.06827893720562361}, {"frequency"=0.4126626626626529, "magnitude"=0.6923975954701067, "weight"=1.0, "phase"=0.0691318766335971}, {"frequency"=0.4129963296629865, "magnitude"=0.6922833802019289, "weight"=1.0, "phase"=0.07004006651785599}, {"frequency"=0.41332999666332015, "magnitude"=0.6923613004671604, "weight"=1.0, "phase"=0.07103157180064934}, {"frequency"=0.4136636636636538, "magnitude"=0.6926481993670456, "weight"=1.0, "phase"=0.07212425933021871}, {"frequency"=0.4139973306639875, "magnitude"=0.6931096403033934, "weight"=1.0, "phase"=0.07329396119255338}, {"frequency"=0.41433099766432113, "magnitude"=0.6936979647063329, "weight"=1.0, "phase"=0.07450568078510078}, {"frequency"=0.4146646646646548, "magnitude"=0.6943653682907756, "weight"=1.0, "phase"=0.07572442149479763}, {"frequency"=0.41499833166498845, "magnitude"=0.6950637580699527, "weight"=1.0, "phase"=0.07691518670858022}, {"frequency"=0.4153319986653221, "magnitude"=0.6957446752098845, "weight"=1.0, "phase"=0.0780429798133857}, {"frequency"=0.41566566566565577, "magnitude"=0.6963592847933929, "weight"=1.0, "phase"=0.07907280419615015}, {"frequency"=0.41599933266598943, "magnitude"=0.6968584338078152, "weight"=1.0, "phase"=0.07996966324381072}, {"frequency"=0.4163329996663231, "magnitude"=0.6971927785335901, "weight"=1.0, "phase"=0.08069856034330347}, {"frequency"=0.41666666666665675, "magnitude"=0.6973129819653453, "weight"=1.0, "phase"=0.0812244988815658}]}, {"frequency point"=[{"frequency"=0.5, "magnitude"=0.0, "weight"=1.0, "phase"=0.0}]}] {"frequency point"."weight" format="%.2f"}
  # "Select Help>>Show Context Help and move the cursor over the VI icon for more information."
  # "freq"
  # "magnitude"
  # "weight"
  # "phase"
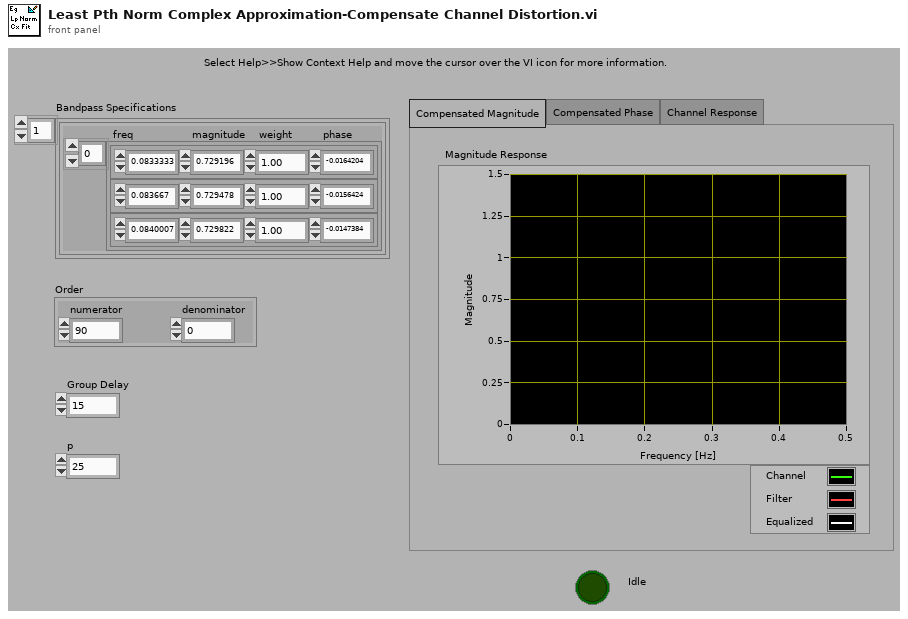
[diagram p1: front panel]
types:
  T1 = enum32{"Compensated Magnitude", "Compensated Phase", "Channel Response"}
  T2 = cluster{"frequency point":cluster{"frequency":dbl, "magnitude":dbl, "weight":dbl, "phase":dbl}[]}[]
  T3 = typedef "NI_DigFilterLicensed.lvlib/DFD Phase Setting.ctl" = cluster{"unwrap? (F)":bool, "degree? (F)":bool}
  T4 = typedef "NI_DigFilterLicensed.lvlib/dfd_Lp Norm Filter Type.ctl" = enum16{"Symmetric", "Antisymmetric", "Differentiator", "Hilbert", "Minimum Phase", "Maximum Phase"}
  T5 = cluster{"frequency point":cluster{"frequency":dbl, "magnitude":dbl, "weight":dbl, "phase":dbl}[]}
  T6 = cluster{"frequency":dbl, "magnitude":dbl, "weight":dbl, "phase":dbl}[]
  T7 = typedef "NI_DigFilterLicensed.lvlib/DFD Filter Obj.ctl" = cluster{"mSRate_Fs":dbl, "mSRate_Version":string, "mSRate_Comments":string, "mSRate_OrgCoef":T8, "mSRate_CurCoef":T8, "mSRate_Quantized?":bool, "mSRate_QCoef":T8, "mSRate_QSettings":T10[], "mSRate_Order":i32, "mSRate_Scaling":cluster{"mSRate_ScaleByPowerOf2?":bool, "mSRate_ScaleType":T12}}
  T8 = typedef "NI_DigFilterLicensed.lvlib/DFD Filter Coef.ctl" = cluster{"type":T9, "gain":dbl, "coef a (k)":dbl[], "coef b (v)":dbl[]}
  T9 = typedef "NI_DigFilterLicensed.lvlib/DFD Filter Structure Type Selector.ctl" = enum16{"Undefined", "FIR Direct Form", "FIR Direct Form Transposed", "FIR Symmetric", "FIR Antisymmetric", "IIR Direct Form I", "IIR Direct Form I Transposed", "IIR Direct Form II", "IIR Direct Form II Transposed", "IIR Cascaded Second Order Sections Form I", "IIR Cascaded Second Order Sections Form I Transposed", "IIR Cascaded Second Order Sections Form II", "IIR Cascaded Second Order Sections Form II Transposed", "Lattice Allpass (basic sections)", "Lattice Allpass (one multiplier sections)", "Lattice Allpass (normalized sections)", "Lattice AR (basic sections)", "Lattice AR (one multiplier sections)", "Lattice AR (normalized sections)", "Lattice MA (minimum phase)", "Lattice MA (maximum phase)", "Lattice ARMA (basic sections)", "Lattice ARMA (one multiplier sections)", "Lattice ARMA (normalized sections)"}
  T10 = typedef "NI_DigFilterLicensed.lvlib/dfd_Internal Quantization Settings.ctl" = cluster{"source":T11, "wl":i16, "iwl":i16, "overflow mode":enum16{"Saturation", "Wrap"}, "rounding mode":enum16{"Nearest", "Truncation"}, "signed?":bool}
  T11 = typedef "NI_DigFilterLicensed.lvlib/dfd_Internal Quantization Srcs.ctl" = u16
  T12 = typedef "NI_DigFilterLicensed.lvlib/DFD Coef Norm Type.ctl" = enum16{"No Norm", "Time Domain 1-Norm", "Time Domain 2-Norm", "Time Domain Inf-Norm"}
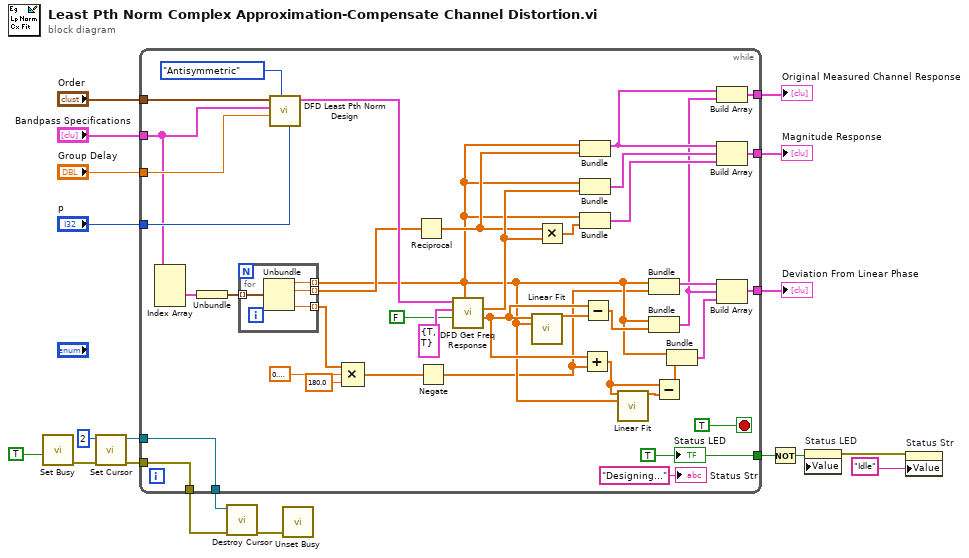
[diagram p0: block diagram]
diagram:
  n1 = call <vilib>:"Set Busy.vi"("disable click? (T)"=TRUE) -> ("error out"=w7:errorcluster)  [unwired: 3 in, 7 out]
  n2 = call-poly <vilib>:"Set Cursor.vi"("error in (no error)"=w7, "icon"=u16 2) -> ("error out"=w5:errorcluster, "previous cursor ID"=w4:refnum<k1>)  [unwired: 1 in, 7 out]
  n3 = while {
    tunnel: "Group Delay" -> [w59]
    tunnel: "Order" -> [w58]
    tunnel: "p" -> [w56]
    tunnel: [w45] -> w19
    tunnel: [w41] -> w18
    tunnel: [w27] -> w17
    tunnel: "Bandpass Specifications" -> [w25]
    tunnel: [w22] -> w15
    tunnel: w5 -> [w21]
    tunnel: [w21] -> w2
    tunnel: [w20] -> w3
    tunnel: w4 -> [w20]
    stop <- TRUE stop-if-true
    w22 = TRUE ("Status")
    n4 = Index Array(array=w25) -> (element #2=w51:T5)  [unwired: 3 in, 2 out]
    n5 = Unbundle(w51) -> ("frequency point"=w52:T6)
    n6 = for {
      tunnel: w52 -> [w63] mode=indexing
      tunnel: [w62] -> w36 mode=indexing
      tunnel: [w61] -> w50 mode=indexing
      tunnel: [w60] -> w40 mode=indexing
      n7 = Unbundle(w63) -> ("frequency"=w62:dbl, "magnitude"=w61:dbl, "phase"=w60:dbl)  [unwired: 1 out]
    }
    n8 = call-poly <vilib>:"DFD Least Pth Norm Design.vi"("p (128)"=w56, "filter type"=dfd_Lp_Norm_Filter_Type."Antisymmetric", "group delay"=w59, "band specs"=w25, "order"=w58) -> ("filter out"=w53:T7)  [unwired: 3 in, 3 out]
    n9 = Compound Arithmetic op=MULTIPLY(w40, 0.3183098861837907, 180.0 ("value")) -> (w31:dbl[])
    n10 = Reciprocal(x=w50) -> (1/x=w44:dbl[])
    n11 = Negate(x=w31) -> (-x=w32:dbl[])
    n12 = call <vilib>:"DFD Get Freq Response.vi"("freq points [Hz]"=w36, "dB on? (T)"=FALSE, "phase view"=T3 {"unwrap? (F)"=TRUE, "degree? (F)"=TRUE}, "filter in"=w53) -> ("phase"=w38:dbl[], "magnitude"=w49:dbl[])  [unwired: 3 in, 3 out]
    n13 = call <vilib>:"Linear Fit.vi"("Y"=w38, "X"=w36) -> ("Best Linear Fit"=w39:dbl[])  [unwired: 4 in, 9 out]
    n14 = Multiply(x=w44, y=w49) -> (x*y=w48:dbl[])
    n15 = Bundle(w36, w44) -> (w28:cluster{dbl[], dbl[]})  [unwired: 1 out]
    n16 = Bundle(w36, "magnitude"=w49) -> (w47:cluster{dbl[], "magnitude":dbl[]})  [unwired: 1 out]
    n17 = Bundle(w36, w48) -> (w46:cluster{dbl[], dbl[]})  [unwired: 1 out]
    n18 = Add(x=w38, y=w32) -> (x+y=w34:dbl[])
    n19 = Subtract(x=w38, y=w39) -> (x-y=w37:dbl[])
    n20 = call <vilib>:"Linear Fit.vi"("Y"=w34, "X"=w36) -> ("Best Linear Fit"=w35:dbl[])  [unwired: 4 in, 9 out]
    n21 = Bundle(w36, w32) -> (w42:cluster{dbl[], dbl[]})  [unwired: 1 out]
    n22 = Bundle(w36, w37) -> (w26:cluster{dbl[], dbl[]})  [unwired: 1 out]
    n23 = Subtract(x=w34, y=w35) -> (x-y=w33:dbl[])
    n24 = Bundle(w36, w33) -> (w43:cluster{dbl[], dbl[]})  [unwired: 1 out]
    n25 = Build Array(w28, w26) -> (w27:cluster{dbl[], dbl[]}[])
    n26 = Build Array(w28, w47, w46) -> (w45:cluster{dbl[], "magnitude":dbl[]}[])
    n27 = Build Array(w42, w26, w43) -> (w41:cluster{dbl[], dbl[]}[])
    "Status LED" <- w22
    "Status Str" <- "Designing..." ("String")
  }
  "Magnitude Response" <- w19
  "Deviation From Linear Phase" <- w18
  "Original Measured Channel Response" <- w17
  n28 = call <vilib>:"Destroy Cursor.vi"("cursor ID"=w3, "error in (no error)"=w2) -> ("error out"=w1:errorcluster)  [unwired: 8 out]
  n29 = call <vilib>:"Unset Busy.vi"("error in (no error)"=w1) -> ()  [unwired: 1 in, 10 out]
  n30 = Not(x=w15) -> (.not. x?=w14:bool)
  n31 = property on="Status LED" class="Bool (strict)"("Value"=w14) -> (error out=w13:errorcluster)  [unwired: 2 in, 1 out]
  n32 = property on="Status Str" class="Str"(error in=w13, "Value"="Idle" ("Boolean Text.Text")) -> ()  [unwired: 1 in, 2 out]
